vi "Synthetic_Jet_Per_Block.vi"() -> (5 "Plug in titles":string[](array[string]), 7 "Plug in values":string[](array[string]))   [LabVIEW 2011]
uses:
  Globals/Meas_global.vi
  Globals/Plug_in_data_global.vi
  <vilib>/Analysis/baseanly.llb/Scale 1D.vi
  <vilib>/Analysis/5stat.llb/RMS (DBL).vi
  <vilib>/Analysis/1siggen.llb/Ramp Pattern by Samples.vi
  <vilib>/Analysis/NI_AALBase.lvlib
  <vilib>/Analysis/NI_AALPro.lvlib
  <vilib>/Analysis/NI_AAL_SigProc.lvlib
panel:
  out "Max Current":dbl format="%0.2f"
  out "RMS Current":dbl format="%0.2f"
  out "RMS Power":dbl format="%0.2f"
  out "Current":dbl[](array[numeric])
  out "RV RMS Pressure":dbl format="%0.2f"
  out "Max Pressure":dbl format="%0.2f"
  out "RMS Dispacement":dbl format="%0.2f"
  out "Max Displacement":dbl format="%0.2f"
  out "Power":dbl[](array[numeric])
  out "Current Plot":cluster{dbl[], dbl[]}[](graph)
  out "RV Pressure":dbl[](array[numeric])=[-14.369666524328046, -57.77058962565634, -87.07652966541758, -117.51006835010423, -142.3114261743131, -158.09199483911908, -155.83679754926837, -151.8902022920296, -142.3114261743131, -120.32906496241762, -88.20412831034297, -49.31359978871612, -12.114469234477319, 29.02544421285115, 67.35217341201532, 101.7323073539407, 128.78305010385122, 147.3826153809706, 157.5310031852989, 162.59938472331393, 149.63781267082135, 136.11244129586606, 102.29610667640338, 72.99016663664214, 42.55081558780641, -5.354689729074237, -48.18600114379076, -84.25753305310417, -116.38246970517886, -138.36483091707433, -158.65579416158175, -165.41557366698484, -160.34719212896982, -149.0712056797162, -122.58426225226835, -92.71452289004439, -56.642990980730964, -17.188663136641456, 24.515049633149694, 61.15038086492581, 97.22191277423924, 132.1658460386273, 151.3292106382094, 160.34418743346322, 160.34418743346322, 155.27580589544817, 136.67624061832876, 106.80650125610484, 74.67575223988108, 33.5358387925526, -1.9718937942981463, -42.553820283313044, -85.38513169802953, -116.38246970517886, -141.74762685185044, -159.78339280650712, -164.28797502205947, -162.03859009635784, -141.18382752938774, -123.71186089719372, -94.40592085743245, -59.46198759304437, -20.007659748954865, 21.70186538498539, 58.3313842526124, 92.14771887207513, 124.27846788829885, 149.63781267082135, 160.34418743346322, 156.9672038628362, 155.27580589544817, 141.75043452049292, 110.18348482673184, 77.49474885219449, 41.987016265343726, 0.2833034955525799, -41.42622163838768, -76.37015490277572, -109.62269019977577, -131.59923904752216, -159.21959348404445, -167.67077095683558, -160.9109914514325, -151.8902022920296, -125.96705818704444, -102.29329900776088, -63.96656980859674, -33.53303112391013, 16.627671482821253, 53.82680203706004, 93.27531751700047, 122.58706992091082, 148.51021402589598, 158.65860183022428, 155.27580589544817, 156.9672038628362, 142.30842147880648, 120.3318726310601, 80.31374546450789, 48.18880881243323, 10.425878935731753, -34.6606297688355, -76.37015490277572, -108.49509155485042, -133.85443633737287, -151.8902022920296, -162.03859009635784, -164.28797502205947, -154.709198904343, -135.54583430476092, -104.54849629761163, -71.85976032307427, -32.96923180144745, 7.0430830009556615, 52.135404069672006, 85.95173868913471, 118.64047466367205, 142.30842147880648, 157.5310031852989, 159.78038811100052, 158.09480250776156, 142.30842147880648, 123.71466856583618, 86.5155380115974, 49.316407457358586, 13.244875548045162, -27.33705094096973, -69.04076371076087, -103.42089765268625, -130.4716404025968, -151.8902022920296, -160.34719212896982, -162.60238941882054, -154.14539958188033, -135.54583430476092, -104.54849629761163, -71.85976032307427, -36.91582705868622, 4.793698075254034, 51.007805424746635, 81.44134410943326, 115.82147805135864, 140.62283587556755, 154.1482072505228, 160.9079867559259, 156.40340454037351, 145.69121741358256, 120.89567195352278, 93.27531751700047, 54.95440068198541]
  out "RV Max Pressure":dbl format="%0.2f"
  out "Max Hot Wire":dbl
  in  "Ring":u16(ring) items=["Pressure", "Velocity"]
  out "RMS Hot Wire":dbl format="%0.2f"
  out "RMS Pressure":dbl format="%0.2f"
  out "Pressure v Frequency":cluster{dbl[], dbl[]}(graph)
  out "Pressure":cluster{dbl[], dbl[]}[](graph)
  out "Displacement":cluster{dbl[], dbl[]}[](graph)
  out "Hot Wire":cluster{dbl[], dbl[]}[](graph)
  out "Input Voltage":dbl[](array[numeric])=[-2.335942353515625, -4.445075804443359, -6.4589520715332025, -8.30833544555664, -9.929101578369139, -11.296158333740234, -12.468054029541014, -13.27053771972656, -13.752864338378906, -13.877860350341795, -13.706862088623046, -13.197119987792966, -12.333764633789063, -11.183243720703125, -9.745557248535155, -8.082506219482422, -6.230334830322265, -4.188578411865234, -2.067363562011719, 0.10821758300781249, 2.266141298828125, 4.396184863281249, 6.422607198486327, 8.238069721679688, 9.855583170166014, 11.26864217529297, 12.397788305664061, 13.200271995849608, 13.694680013427734, 13.847556176757811, 13.67051721557617, 13.127318933105467, 12.284873692626952, 11.125059395751952, 9.687837592773436, 8.003411781005859, 6.15077572265625, 4.139687470703125, 2.006391221923828, -0.14781514038085936, -2.321072939453125, -4.453904519042968, -6.44965868774414, -8.280919963378906, -9.916555510253906, -11.332867199707032, -12.452719946289061, -13.252415621337889, -13.737530255126952, -13.89923513305664, -13.710114772949218, -13.191079288330076, -12.333764633789063, -11.186031735839844, -9.7520626171875, -8.079718204345703, -6.215000747070311, -4.203912495117187, -2.088738344726562, 0.09613618408203123, 2.2508072155761716, 4.374810080566406, 6.367311564941406, 8.235281706542969, 9.874169937744139, 11.26864217529297, 12.38245422241211, 13.197483980712889, 13.700720712890623, 13.85638489135742, 13.661223831787108, 13.136147647705076, 12.263498909912107, 11.116230681152343, 9.681796893310546, 8.027574578857422, 6.160069106445311, 4.139687470703125, 2.021725305175781, -0.1357337414550781, -2.321072939453125, -4.426489036865234, -6.452911372070313, -8.280919963378906, -9.925848894042968, -11.308239732666014, -12.419263764648436, -13.261244335937498, -13.752864338378906, -13.914569216308593, -13.72544885620117, -13.182250573730467, -12.343058017578123, -11.198577803955077, -9.760891331787109, -8.107133686523436, -6.22382946166992, -4.215993894042969, -2.107325112304687, 0.08684280029296874, 2.2415138317871093, 4.365516696777344, 6.382645648193359, 8.207866224365233, 9.855583170166014, 11.222639925537107, 12.37966620727539, 13.200271995849608, 13.67655791503906, 13.841050808105468, 13.62451496582031, 13.118025549316405, 12.27279229370117, 11.131100095214844, 9.705959691162109, 8.048949361572266, 6.181443889160155, 4.1824370361328125, 2.040312072753906, -0.1357337414550781, -2.3024861718749996, -4.414407637939453, -6.422243205566406, -8.24142308227539, -9.907726795654296, -11.314280432128905, -12.452719946289061, -13.26449702026367, -13.746823638916014, -13.89923513305664, -13.700821389160156, -13.20037267211914, -12.357927431640622, -11.195325119628905, -9.733475849609373, -8.115962401123046, -6.245204244384766, -4.2220345935058585, -2.091991029052734, 0.08405478515624998, 2.226179748535156, 4.3473945983886715, 6.331067368164062, 8.19253214111328, 9.840249086914062, 11.237974008789063, 12.367120139160155, 13.182149897460938, 13.691891998291014, 13.828969409179685, 13.657971147460938, 13.139400332031247, 12.278832993164063, 11.131100095214844, 9.6971309765625, 8.048949361572266, 6.190272603759766, 4.161062253417969, 2.055181486816406, -0.11761164306640623, -2.284364073486328, -4.393032855224609, -6.410161806640624, -8.265585880126952, -9.916555510253906, -11.314280432128905, -12.431345163574218, -13.261244335937498, -13.761693052978515, -13.908528516845703, -13.716155472412108, -13.20641337158203, -12.343058017578123, -11.207406518554686, -9.785518798828125, -8.115962401123046, -6.2331228454589835, -4.23411599243164, -2.110113127441406, 0.05663930297851562, 2.2168863647460935, 4.35018261352539, 6.345936782226563, 8.19857284057617, 9.822126988525389, 11.241226693115234, 12.361079439697264, 13.227687478027343, 13.682598614501952, 13.838262792968749, 13.645889748535156, 13.136147647705076, 12.290914392089842, 11.143646163330077, 9.727334473876951, 8.027574578857422, 6.187484588623047, 4.176396336669922, 2.052393471679687, -0.1264403576660156, -2.2718180053710935, -4.389780170898437, -6.398080407714843, -8.24746378173828, -9.901221427001953, -11.308239732666014, -12.455972630615232, -13.246374921874999, -13.761693052978515, -13.89923513305664, -13.716155472412108, -13.20641337158203, -12.361180115966796, -11.207406518554686, -9.773437399902342, -8.119215085449218, -6.263791011962891, -4.252702760009765, -2.11661849609375, 0.0320118359375, 2.2140983496093747, 4.319979116210937, 6.339896082763671, 8.1804507421875, 9.843501771240234, 11.231933309326172, 12.364332124023436, 13.178897213134764, 13.688639313964844, 13.847556176757811, 13.636596364746092, 13.139400332031247, 12.306248475341796, 11.149686862792967, 9.721293774414061, 8.07357682861328, 6.220940770263671, 4.188477735595702, 2.0644748706054687, -0.09623686035156248, -2.2690299902343747, -4.389780170898437, -6.394827723388671, -8.244211097412109, -9.879846644287108, -11.302199033203124, -12.422051779785155, -13.252415621337889, -13.749611654052734, -13.902487817382811, -13.722196171874998, -13.20037267211914, -12.357927431640622, -11.186031735839844, -9.791559498291015, -8.115962401123046, -6.273084395751952, -4.2373686767578125, -2.1347405944824214, 0.041305219726562495, 2.208057650146484, 4.313473747558593, 6.3371080676269536, 8.167904674072265, 9.831420372314453, 11.235185993652344, 12.38245422241211, 13.197483980712889, 13.691891998291014, 13.835010108642576, 13.661223831787108, 13.15148173095703, 12.309036490478515, 11.158980246582031, 9.736627857666015, 8.085658227539062, 6.16889782104492, 4.209852518310547, 2.089102337646484, -0.09902487548828123, -2.262989290771484, -4.386992155761718, -6.394827723388671, -8.244211097412109, -9.879846644287108, -11.28082425048828, -12.428092479248045, -13.239869553222654, -13.73427757080078, -13.902487817382811, -13.73148955566406, -13.203625356445311, -12.370473499755859, -11.21669990234375, -9.797600197753905, -8.101092987060547, -6.281913110351562, -4.268036843261719, -2.128699895019531, 0.03526452026367187, 2.208057650146484, 4.316726431884765, 6.312480600585937, 8.155823275146483, 9.831420372314453, 11.241226693115234, 12.345745356445313, 13.166815814208983, 13.685386629638671, 13.853596876220703, 13.673305230712888, 13.148693715820311, 12.300207775878905, 11.155727562255858, 9.727334473876951, 8.113073709716796, 6.233022169189453, 4.213105202636719, 2.089102337646484, -0.0776500927734375, -2.2355738085937498, -4.374910756835937, -6.38274632446289, -8.222836314697265, -9.877058629150389, -11.296158333740234, -12.3918482824707, -13.243122237548828, -13.740318270263671, -13.914569216308593, -13.737530255126952, -13.20641337158203, -12.373261514892578, -11.244115384521482, -9.81618696533203, -8.149883251953124, -6.273084395751952, -4.240621361083984, -2.140781293945312, 0.02597113647460937, 2.1955115820312496, 4.29209896484375, 6.315733284912108, 8.159075959472656, 9.824915003662108, 11.201265142822265, 12.355038740234374, 13.176109197998045, 13.664476516113279, 13.835010108642576, 13.664476516113279, 13.160775114746093, 12.288126376953123, 11.16502094604492, 9.745921241455077, 8.094951611328124, 6.218152755126952, 4.23122730102539, 2.110477120361328, -0.08415546142578124, -2.2323211242675782, -4.362364688720703, -6.3613715417480465, -8.214007600097656, -9.861724545898436, -11.284076934814454, -12.413223065185546, -13.243122237548828, -13.755652353515623, -13.908528516845703, -13.722196171874998, -13.225000139160155, -12.370473499755859, -11.250156083984375, -9.82501567993164, -8.158711966552733, -6.303287893066406, -4.28615894165039, -2.186783543701172, 0.010637053222656246, 2.1746014685058594, 4.29209896484375, 6.294358502197265, 8.149782575683593, 9.76125532470703, 11.213811210937498, 12.361079439697264, 13.178897213134764, 13.673305230712888, 13.838262792968749, 13.673305230712888, 13.154734415283203, 12.321582558593748, 11.179890360107422, 9.748709256591797, 8.100992310791016, 6.242315552978514, 4.215893217773437, 2.1039717517089844, -0.0627806787109375, -2.2202397253417967, -4.328908507080078, -6.367412241210937, -8.161964650878906, -9.871017929687499, -11.265490167236328, -12.397888981933594, -13.233828853759764, -13.712902788085938, -13.908528516845703, -13.73427757080078, -13.218494770507812, -12.373261514892578, -11.238074685058592, -9.828268364257811, -8.168005350341796, -6.32187466064453, -4.28615894165039, -2.186783543701172, -0.016778428955078126, 2.159267385253906, 4.28327025024414, 6.309692585449218, 8.137701176757812, 9.797499521484374, 11.204517827148436, 12.3369166418457, 13.166815814208983, 13.67934593017578, 13.838262792968749, 13.661223831787108, 13.15752243041992, 12.321582558593748, 11.204517827148436, 9.77612473876953, 8.140489191894531, 6.220940770263671, 4.237268000488281, 2.1378926025390625, -0.05627531005859375, -2.2202397253417967, -4.3502832897949215, -6.343249443359374, -8.201461531982421, -9.861724545898436, -11.256196783447265, -12.397888981933594, -13.237081538085938, -13.749611654052734, -13.895982448730468, -13.728236871337888, -13.21245407104492, -12.38255489868164, -11.247368068847656, -9.861724545898436, -8.18938013305664, -6.309328592529297, -4.304281040039061, -2.177490159912109, -0.02003111328125, 2.1499740014648436, 4.258642783203125, 6.285065118408203, 8.13444849243164, 9.77612473876953, 11.195224443359375, 12.321582558593748, 13.182149897460938, 13.673305230712888, 13.822928709716795, 13.664476516113279, 13.172856513671874, 12.3369166418457, 11.22589260986328, 9.779377423095703, 8.113073709716796, 6.26973103515625, 4.261895467529296, 2.1499740014648436, -0.03211251220703125, -2.198864942626953, -4.328908507080078, -6.327915360107421, -8.171258034667968, -9.846390462646484, -11.268742851562498, -12.397888981933594, -13.221747454833983, -13.737530255126952, -13.895982448730468, -13.758905037841796, -13.237081538085938, -12.406717696533203, -11.262702152099608, -9.837561748046875, -8.186127448730469, -6.33674407470703, -4.313574423828125, -2.183530859375, -0.04140589599609375, 2.143933302001953, 4.255854768066406, 6.28181243408203, 8.125155108642577, 9.788670806884765, 11.179890360107422, 12.324370573730468, 13.15752243041992, 13.682598614501952, 13.85034419189453, 13.67051721557617, 13.163563129882812, 12.330411273193358, 11.201265142822265, 9.785418122558593, 8.125155108642577, 6.26694302001953, 4.264683482666015, 2.1467213171386716, -0.016778428955078126, -2.183530859375, -4.310786408691406, -6.327915360107421, -8.161964650878906, -9.828268364257811, -11.244115384521482, -12.38255489868164, -13.221747454833983, -13.72544885620117, -13.908528516845703, -13.706862088623046, -13.233828853759764, -12.400676997070313, -11.262702152099608, -9.852431162109374, -8.180086749267577, -6.33674407470703, -4.325655822753906, -2.208158326416015, -0.04140589599609375, 2.131851903076172, 4.261895467529296, 6.26694302001953, 8.137701176757812, 9.779377423095703, 11.192436428222656, 12.318329874267578, 13.170068498535155, 13.688639313964844, 13.838262792968749, 13.67655791503906, 13.172856513671874, 12.348998040771484, 11.210558526611328, 9.794711506347655, 8.13444849243164, 6.279024418945312, 4.28327025024414, 2.1653080847167967, -0.016778428955078126, -2.180278175048828, -4.304281040039061, -6.339996759033203, -8.161964650878906, -9.822227664794921, -11.238074685058592, -12.38255489868164, -13.215706755371093, -13.728236871337888, -13.89923513305664, -13.737530255126952, -13.243122237548828, -12.403929681396484, -11.277571566162107, -9.846390462646484, -8.18938013305664, -6.349290142822265, -4.353535974121093, -2.2295331091308594, -0.050234610595703125, 2.12859921875, 4.2800175659179684, 6.233022169189453, 8.103780325927733, 9.773336723632811, 11.192436428222656, 12.318329874267578, 13.160775114746093, 13.67655791503906, 13.847556176757811, 13.688639313964844, 13.184937912597654, 12.33970465698242, 11.204517827148436, 9.797499521484374, 8.146529891357421, 6.2911058178710935, 4.286058265380859, 2.1653080847167967, -0.013525744628906253, -2.1714494604492183, -4.28615894165039, -6.297247193603514, -8.168005350341796, -9.822227664794921, -11.22878130126953, -12.361180115966796, -13.203625356445311, -13.72544885620117, -13.917357231445312, -13.749611654052734, -13.218494770507812, -12.397888981933594, -11.256196783447265, -9.871017929687499, -8.214007600097656, -6.352078157958983, -4.328908507080078, -2.2230277404785155, -0.09623686035156248, 2.1039717517089844, 4.225186601562499, 6.2455682373046875, 8.094951611328124, 9.764043339843749, 11.16502094604492, 12.306248475341796, 13.15148173095703, 13.67051721557617, 13.84430349243164, 13.682598614501952, 13.184937912597654, 12.318329874267578, 11.231933309326172, 9.816086289062499, 8.161863974609375, 6.297146517333983, 4.2800175659179684, 2.2168863647460935, -0.026071812744140627, -2.162156076660156, -4.28615894165039, -6.291206494140624, -8.161964650878906, -9.81618696533203, -11.21995258666992, -12.373261514892578, -13.227788154296874, -13.740318270263671, -13.91131653198242, -13.737530255126952, -13.215706755371093, -12.419263764648436, -11.286864949951172, -9.861724545898436, -8.20750223144531, -6.364624226074218, -4.383739471435547, -2.2536959069824216, -0.07160939331054687, 2.0979310522460937, 4.200559134521484, 6.239527537841796, 8.079617528076172, 9.754749956054686, 11.16176826171875, 12.315541859130859, 13.139400332031247, 13.661223831787108, 13.826181394042967, 13.657971147460938, 13.188190596923828, 12.358291424560546, 11.231933309326172, 9.816086289062499, 8.173945373535155, 6.315733284912108, 4.313473747558593, 2.1927235668945313, 0.013889737548828125, -2.162156076660156, -4.270824858398437, -6.3004998779296875, -8.143842552490234, -9.803640897216797, -11.21995258666992, -12.373261514892578, -13.215706755371093, -13.716155472412108, -13.874607666015624, -13.73427757080078, -13.243122237548828, -12.413223065185546, -11.284076934814454, -9.879846644287108, -8.226088999023437, -6.38274632446289, -4.368405388183593, -2.2416145080566405, -0.07486207763671875, 2.0798089538574214, 4.207064503173828, 6.230234154052734, 8.06753612915039, 9.739880541992186, 11.16176826171875, 12.300207775878905, 13.160775114746093, 13.655183132324218, 13.838262792968749, 13.67934593017578, 13.182149897460938, 12.370372823486326, 11.207770511474608, 9.824915003662108, 8.161863974609375, 6.315733284912108, 4.316726431884765, 2.1955115820312496, 0.02271845214843749, -2.13148791015625, -4.258743459472656, -6.266579027099609, -8.13733718383789, -9.791559498291015, -11.210659202880858, -12.361180115966796, -13.246374921874999, -13.719408156738279, -13.895982448730468, -13.746823638916014, -13.246374921874999, -12.43459784790039, -11.292905649414063, -9.88914002807617, -8.25350448120117, -6.38274632446289, -4.383739471435547, -2.2657773059082027, -0.10831825927734373, 2.0798089538574214, 4.203811818847656, 6.21490007080078, 8.07357682861328, 9.733375173339843, 11.158980246582031, 12.32762325805664, 13.154734415283203, 13.661223831787108, 13.838262792968749, 13.682598614501952, 13.20352468017578, 12.370372823486326, 11.235185993652344, 9.818874304199218, 8.173945373535155, 6.32781468383789, 4.338101214599609, 2.2140983496093747, 0.05338661865234373, -2.1226591955566403, -4.249450075683593, -6.251709613037109, -8.119215085449218, -9.779478099365233, -11.213911887207031, -12.363968131103515, -13.20037267211914, -13.722196171874998, -13.89923513305664, -13.752864338378906, -13.246374921874999, -12.425304464111326, -11.311492416992186, -9.886352012939453, -8.24746378173828, -6.416202506103516, -4.389780170898437, -2.3057388562011716, -0.09902487548828123, 2.0677275549316403, 4.170355637207031, 6.196777972412109, 8.054990061035156, 9.730587158203125, 11.143646163330077, 12.306248475341796, 13.127318933105467, 13.664476516113279, 13.835010108642576, 13.691891998291014, 13.21235339477539, 12.364332124023436, 11.244014708251953, 9.852795155029296, 8.19857284057617, 6.345936782226563, 4.3441419140625, 2.2233917333984374, 0.04734591918945312, -2.1226591955566403, -4.243409376220702, -6.266579027099609, -8.107133686523436, -9.794812182617186, -11.213911887207031, -12.33655264892578, -13.197119987792966, -13.719408156738279, -13.91131653198242, -13.758905037841796, -13.237081538085938, -12.416011080322264, -11.302199033203124, -9.916555510253906, -8.250251796874998, -6.3613715417480465, -4.420448337402344, -2.2931927880859373, -0.1264403576660156, 2.0491407873535157, 4.17314365234375, 6.181443889160155, 8.052202045898436, 9.718505759277342, 11.140393479003905, 12.300207775878905, 13.133359632568357, 13.657971147460938, 13.862425590820312, 13.685386629638671, 13.160775114746093, 12.364332124023436, 11.247267392578124, 9.855583170166014, 8.161863974609375, 6.349189466552733, 4.334848530273437, 2.2382611474609373, 0.05942731811523437, -2.1040724279785157, -4.209953194580078, -6.248456928710937, -8.109921701660156, -9.760891331787109, -11.189284420166015, -12.349098717041013, -13.185038588867187, -13.722196171874998, -13.902487817382811, -13.758905037841796, -13.26449702026367, -12.422051779785155, -11.311492416992186, -9.919808194580078, -8.265585880126952, -6.428748574218749, -4.423701021728515, -2.2871520886230465, -0.1264403576660156, 2.052393471679687, 4.176396336669922, 6.172150505371094, 8.042908662109374, 9.70317167602539, 11.146434178466794, 12.284873692626952, 13.114772864990234, 13.643101733398437, 13.853596876220703, 13.688639313964844, 13.188190596923828, 12.373160838623045, 11.259348791503905, 9.849542470703124, 8.204613540039063, 6.367311564941406, 4.365516696777344, 2.2568479150390623, 0.07476140136718748, -2.0859503295898434, -4.2067005102539055, -6.2331228454589835, -8.107133686523436, -9.76693203125, -11.186031735839844, -12.318430550537107, -13.191079288330076, -13.722196171874998, -13.91131653198242, -13.746823638916014, -13.26449702026367, -12.440638547363282, -11.317533116455076, -9.929101578369139, -8.271626579589844, -6.428748574218749, -4.435782420654297, -2.2931927880859373, -0.14781514038085936, 2.0310186889648434, 4.155021553955078, 6.1628571215820305, 8.030827263183593, 9.693878292236327, 11.076269130859373, 12.263498909912107, 13.120813564453124, 13.655183132324218, 13.859637575683593, 13.688639313964844, 13.20352468017578, 12.370372823486326, 11.253308092041014, 9.861623869628906, 8.216694938964844, 6.367311564941406, 4.362264012451171, 2.2415138317871093, 0.09009548461914062, -2.082697645263672, -4.209953194580078, -6.22382946166992, -8.088546918945312, -9.730687834472656, -11.183243720703125, -12.321683234863281, -13.188291273193357, -13.712902788085938, -13.917357231445312, -13.752864338378906, -13.26728503540039, -12.446679246826172, -11.32682650024414, -9.94397099243164, -8.286960662841796, -6.440829973144531, -4.429741721191406, -2.321072939453125, -0.16036120849609373, 2.0189372900390623, 4.127606071777343, 6.156816422119141, 8.018281195068358, 9.70317167602539, 11.11297799682617, 12.269539609375, 13.127318933105467, 13.657971147460938, 13.85034419189453, 13.703973397216796, 13.197483980712889, 12.38245422241211, 11.256560776367186, 9.867664569091797, 8.238069721679688, 6.37985763305664, 4.365516696777344, 2.2568479150390623, 0.09009548461914062, -2.067363562011719, -4.182537712402343, -6.236375529785155, -8.073212835693358, -9.760891331787109, -11.171162321777343, -12.333764633789063, -13.182250573730467, -13.704074073486328, -13.91131653198242, -13.749611654052734, -13.26728503540039, -12.43459784790039, -11.335655214843749, -9.956517060546874, -8.302294746093748, -6.452911372070313, -4.445075804443359, -2.321072939453125, -0.16640190795898435, 1.9943098229980465, 4.133646771240234, 6.184231904296874, 8.024786563720703, 9.678544208984373, 11.11297799682617, 12.263498909912107, 13.127318933105467, 13.661223831787108, 13.838262792968749, 13.688639313964844, 13.20352468017578, 12.397788305664061, 11.277935559082032, 9.916454833984375, 8.256656489257812, 6.388686347656249, 4.386891479492187, 2.2721819982910154, 0.10821758300781249]
  out "Displacement":dbl[](array[numeric])=[-0.04333556876627609, -0.0421144060872396, -0.0457758823242187, -0.04516630688476564, -0.02685490209960939, -0.018920362386067757, -0.032349128255208304, -0.02990680289713543, -0.009764659993489633, -0.0030512829589843804, -0.006714770996093744, -0.011597409912109335, 0.017088848144531266, 0.014038959147135377, 0.01892159806315108, 0.01892159806315108, 0.03112718945312498, 0.038452153727213556, 0.03784257828776039, 0.03784257828776039, 0.03967331640625005, 0.04272521720377609, 0.04699626888020836, 0.040282891845703106, 0.02441381241861984, 0.031738776692708304, 0.031738776692708304, 0.02929645133463543, 0.003662094075520872, 0.003662094075520872, 0.006104419433593744, 0.0048832567545572525, -0.014649310709635377, -0.017089624267578096, -0.017699199707031266, -0.02441458854166667, -0.037231767171224006, -0.039672080729166614, -0.039672080729166614, -0.039062505289713556, -0.04150483064778643, -0.04882778312174474, -0.0457758823242187, -0.04516630688476564, -0.02868564021809894, -0.030518390136718754, -0.03173754101562498, -0.02624532666015622, -0.010376247233072955, -0.009155084554036463, -0.007933921874999972, -0.008545509114583294, 0.018310010823567757, 0.019531173502604138, 0.020140748942057307, 0.017088848144531266, 0.03417909025065102, 0.03600982836914057, 0.035400252929687515, 0.035400252929687515, 0.03967331640625005, 0.038452153727213556, 0.04089447908528643, 0.04272521720377609, 0.035400252929687515, 0.028686875895182262, 0.028686875895182262, 0.029908038574218754, 0.008544732991536463, 0.007935157552083294, 0.0030525186360677026, 0.003662094075520872, -0.02136268774414063, -0.018310786946614588, -0.01953194962565108, -0.017699199707031266, -0.04028366796875005, -0.0421144060872396, -0.040893243408203106, -0.039062505289713556, -0.04455471964518232, -0.04516630688476564, -0.0506585212402344, -0.04699704500325519, -0.02624532666015622, -0.02380300130208335, -0.02258385042317712, -0.030518390136718754, -0.012206985351562505, -0.007933921874999972, -0.008545509114583294, -0.0054936083170572525, 0.015258110026041716, 0.015869697265625038, 0.017700435384114588, 0.01892159806315108, 0.03600982836914057, 0.03600982836914057, 0.03112718945312498, 0.03600982836914057, 0.03784257828776039, 0.0415040545247396, 0.04089447908528643, 0.038452153727213556, 0.030517614013671923, 0.02075233618164063, 0.033569514811197965, 0.030517614013671923, 0.0030525186360677026, 0.0024409313964843804, -0.0030512829589843804, -0.0012205448404948305, -0.016480048828125038, -0.018310786946614588, -0.018920362386067757, -0.017089624267578096, -0.03662017993164057, -0.03173754101562498, -0.039062505289713556, -0.039672080729166614, -0.04516630688476564, -0.0457758823242187, -0.04516630688476564, -0.039672080729166614, -0.02807606477864588, -0.02807606477864588, -0.02868564021809894, -0.031127965576171923, -0.008545509114583294, -0.007933921874999972, -0.004272445638020872, -0.012206985351562505, 0.016479272705078096, 0.017700435384114588, 0.028686875895182262, 0.014648534586588546, 0.03417909025065102, 0.03600982836914057, 0.038452153727213556, 0.03967331640625005, 0.037230991048177065, 0.04089447908528643, 0.032959939371744795, 0.039061729166666614, 0.02746571321614588, 0.026856137776692712, 0.028686875895182262, 0.02929645133463543, 0.006104419433593744, 0.0024409313964843804, 0.0024409313964843804, 0.005492832194010422, -0.018920362386067757, -0.020141525065104138, -0.020141525065104138, -0.020751100504557307, -0.037231767171224006, -0.04333556876627609, -0.037231767171224006, -0.037231767171224006, -0.0421144060872396, -0.042723981526692656, -0.0457758823242187, -0.04699704500325519, -0.03173754101562498, -0.027466489339192712, -0.029297227457682262, -0.029297227457682262, -0.013428148030598996, -0.006714770996093744, -0.008545509114583294, -0.006714770996093744, 0.014038959147135377, 0.015258110026041716, 0.017700435384114588, 0.018310010823567757, 0.036621415608724006, 0.035400252929687515, 0.035400252929687515, 0.03417909025065102, 0.042113629964192656, 0.04089447908528643, 0.04272521720377609, 0.03784257828776039, 0.025025399658203162, 0.02929645133463543, 0.03234835213216147, 0.039061729166666614, 0.005492832194010422, 0.0030525186360677026, 0.0006101932779948305, 0.005492832194010422, -0.017089624267578096, -0.017089624267578096, -0.01953194962565108, -0.02380300130208335, -0.039672080729166614, -0.040893243408203106, -0.04028366796875005, -0.04333556876627609, -0.040893243408203106, -0.04699704500325519, -0.040893243408203106, -0.04333556876627609, -0.029297227457682262, -0.030518390136718754, -0.034179866373697965, -0.02685490209960939, -0.011597409912109335, -0.006714770996093744, -0.006103183756510422, -0.009764659993489633, 0.014038959147135377, 0.020140748942057307, 0.02258307430013018, 0.02075233618164063, 0.03112718945312498, 0.034790677490234345, 0.037230991048177065, 0.030517614013671923, 0.04089447908528643, 0.038452153727213556, 0.040282891845703106, 0.038452153727213556, 0.033569514811197965, 0.02807528865559894, 0.031738776692708304, 0.026856137776692712, 0.003662094075520872, 0.001831355957031211, -0.0054936083170572525, 6.178385416610865e-07, -0.014649310709635377, -0.017699199707031266, -0.01953194962565108, -0.017699199707031266, -0.035401029052734345, -0.04150483064778643, -0.040893243408203106, -0.03662017993164057, -0.04699704500325519, -0.0457758823242187, -0.04882778312174474, -0.04455471964518232, -0.030518390136718754, -0.02685490209960939, -0.02868564021809894, -0.030518390136718754, -0.010376247233072955, -0.006714770996093744, -0.006714770996093744, -0.008545509114583294, 0.015869697265625038, 0.02197349886067712, 0.020140748942057307, 0.02197349886067712, 0.03417909025065102, 0.039061729166666614, 0.03600982836914057, 0.036621415608724006, 0.03784257828776039, 0.038452153727213556, 0.036621415608724006, 0.036621415608724006, 0.03112718945312498, 0.03234835213216147, 0.031738776692708304, 0.032959939371744795, 0.0048832567545572525, 0.0006101932779948305, 0.0030525186360677026, 0.00427166951497393, -0.014649310709635377, -0.018310786946614588, -0.016480048828125038, -0.018920362386067757, -0.04516630688476564, -0.036010604492187515, -0.036010604492187515, -0.042723981526692656, -0.04760662044270836, -0.04760662044270836, -0.04882778312174474, -0.04638746956380213, -0.03173754101562498, -0.02990680289713543, -0.034179866373697965, -0.02685490209960939, -0.009764659993489633, -0.006714770996093744, -0.012206985351562505, -0.009764659993489633, 0.015869697265625038, 0.02075233618164063, 0.018310010823567757, 0.02563497509765622, 0.03600982836914057, 0.033569514811197965, 0.040282891845703106, 0.036621415608724006, 0.04333479264322915, 0.03784257828776039, 0.037230991048177065, 0.037230991048177065, 0.03417909025065102, 0.032959939371744795, 0.029908038574218754, 0.026856137776692712, 0.00427166951497393, 0.0067139948730469134, 0.003662094075520872, 0.003662094075520872, -0.018920362386067757, -0.02136268774414063, -0.020751100504557307, -0.013428148030598996, -0.03662017993164057, -0.04028366796875005, -0.040893243408203106, -0.04028366796875005, -0.039672080729166614, -0.0457758823242187, -0.04699704500325519, -0.04821820768229168, -0.031127965576171923, -0.03295870369466147, -0.02136268774414063, -0.02807606477864588, -0.010985822672526013, -0.012206985351562505, -0.012206985351562505, -0.0073243464355469134, 0.016479272705078096, 0.014038959147135377, 0.014648534586588546, 0.016479272705078096, 0.036621415608724006, 0.04455595532226564, 0.037230991048177065, 0.037230991048177065, 0.040282891845703106, 0.039061729166666614, 0.0415040545247396, 0.03600982836914057, 0.03234835213216147, 0.02258307430013018, 0.03112718945312498, 0.02807528865559894, 0.001831355957031211, -0.0006109694010416611, 0.0024409313964843804, 0.006104419433593744, -0.0219722631835938, -0.018310786946614588, -0.020141525065104138, -0.01953194962565108, -0.04150483064778643, -0.039062505289713556, -0.0421144060872396, -0.042723981526692656, -0.04455471964518232, -0.04394514420572915, -0.04516630688476564, -0.04394514420572915, -0.030518390136718754, -0.03295870369466147, -0.02868564021809894, -0.029297227457682262, -0.014037723470052055, -0.010376247233072955, -0.007933921874999972, -0.012206985351562505, 0.018310010823567757, 0.014648534586588546, 0.017700435384114588, 0.014648534586588546, 0.03234835213216147, 0.03600982836914057, 0.03112718945312498, 0.03784257828776039, 0.037230991048177065, 0.040282891845703106, 0.03784257828776039, 0.040282891845703106, 0.0213619116210938, 0.03112718945312498, 0.032959939371744795, 0.02807528865559894, 0.0048832567545572525, 0.0012197687174478888, 0.003662094075520872, 0.0006101932779948305, -0.016480048828125038, -0.02441458854166667, -0.018920362386067757, -0.01953194962565108, -0.036010604492187515, -0.04516630688476564, -0.04455471964518232, -0.0421144060872396, -0.04394514420572915, -0.04150483064778643, -0.04882778312174474, -0.037231767171224006, -0.035401029052734345, -0.025635751220703162, -0.02807606477864588, -0.02685490209960939, -0.006714770996093744, -0.011597409912109335, -0.007933921874999972, -0.007933921874999972, 0.017700435384114588, 0.016479272705078096, 0.016479272705078096, 0.014648534586588546, 0.03600982836914057, 0.038452153727213556, 0.035400252929687515, 0.03112718945312498, 0.038452153727213556, 0.037230991048177065, 0.04455595532226564, 0.038452153727213556, 0.030517614013671923, 0.02929645133463543, 0.02807528865559894, 0.030517614013671923, 0.007935157552083294, 0.0024409313964843804, -0.0006109694010416611, 6.178385416610865e-07, -0.016480048828125038, -0.014649310709635377, -0.016480048828125038, -0.014037723470052055, -0.04516630688476564, -0.04394514420572915, -0.032349128255208304, -0.04150483064778643, -0.04333556876627609, -0.04882778312174474, -0.04638746956380213, -0.04760662044270836, -0.029297227457682262, -0.02685490209960939, -0.030518390136718754, -0.030518390136718754, -0.013428148030598996, -0.0030512829589843804, -0.0073243464355469134, -0.0054936083170572525, 0.014648534586588546, 0.018310010823567757, 0.012817796468098996, 0.018310010823567757, 0.035400252929687515, 0.038452153727213556, 0.034790677490234345, 0.034790677490234345, 0.04272521720377609, 0.036621415608724006, 0.042113629964192656, 0.038452153727213556, 0.02624455053710939, 0.02746571321614588, 0.02563497509765622, 0.03234835213216147, 0.005492832194010422, -0.0018301202799478888, -0.0006109694010416611, 0.005492832194010422, -0.015258886149088546, -0.009764659993489633, -0.02258385042317712, -0.0219722631835938, -0.037231767171224006, -0.040893243408203106, -0.037841342610677065, -0.040893243408203106, -0.04333556876627609, -0.04638746956380213, -0.042723981526692656, -0.0421144060872396, -0.029297227457682262, -0.033570290934244795, -0.02990680289713543, -0.02807606477864588, -0.010376247233072955, -0.007933921874999972, -0.011597409912109335, -0.010376247233072955, 0.012817796468098996, 0.017700435384114588, 0.018310010823567757, 0.019531173502604138, 0.029908038574218754, 0.03784257828776039, 0.037230991048177065, 0.034790677490234345, 0.03784257828776039, 0.0415040545247396, 0.0415040545247396, 0.0415040545247396, 0.032959939371744795, 0.025025399658203162, 0.029908038574218754, 0.026856137776692712, 0.006104419433593744, 0.0030525186360677026, 0.0006101932779948305, -0.0012205448404948305, -0.015258886149088546, -0.017089624267578096, -0.018310786946614588, -0.02136268774414063, -0.039062505289713556, -0.0421144060872396, -0.039672080729166614, -0.03662017993164057, -0.04455471964518232, -0.0457758823242187, -0.04821820768229168, -0.040893243408203106, -0.030518390136718754, -0.025635751220703162, -0.027466489339192712, -0.02868564021809894, -0.010985822672526013, -0.008545509114583294, -0.0006109694010416611, -0.009764659993489633, 0.012817796468098996, 0.015258110026041716, 0.0213619116210938, 0.0213619116210938, 0.037230991048177065, 0.034790677490234345, 0.03600982836914057, 0.033569514811197965, 0.0415040545247396, 0.04333479264322915, 0.039061729166666614, 0.04089447908528643, 0.030517614013671923, 0.03234835213216147, 0.030517614013671923, 0.031738776692708304, 0.0067139948730469134, 6.178385416610865e-07, 0.0012197687174478888, 0.0006101932779948305, -0.013428148030598996, -0.018920362386067757, -0.01953194962565108, -0.02258385042317712, -0.03662017993164057, -0.039672080729166614, -0.037231767171224006, -0.04333556876627609, -0.04699704500325519, -0.04699704500325519, -0.04821820768229168, -0.0421144060872396, -0.03173754101562498, -0.030518390136718754, -0.031127965576171923, -0.02685490209960939, -0.009764659993489633, -0.0054936083170572525, -0.010985822672526013, -0.009764659993489633, 0.015869697265625038, 0.017088848144531266, 0.0213619116210938, 0.01892159806315108, 0.033569514811197965, 0.03234835213216147, 0.03600982836914057, 0.036621415608724006, 0.042113629964192656, 0.04577711800130213, 0.035400252929687515, 0.03784257828776039, 0.03112718945312498, 0.032959939371744795, 0.02807528865559894, 0.02807528865559894, 0.006104419433593744, 0.003662094075520872, 0.005492832194010422, 0.0067139948730469134, -0.018920362386067757, -0.0219722631835938, -0.02258385042317712, -0.018920362386067757, -0.03845292985026039, -0.0421144060872396, -0.04394514420572915, -0.04394514420572915, -0.04333556876627609, -0.04516630688476564, -0.04394514420572915, -0.0506585212402344, -0.03173754101562498, -0.029297227457682262, -0.02380300130208335, -0.025635751220703162, -0.012816560791015674, -0.010985822672526013, -0.010376247233072955, -0.002441707519531211, 0.017700435384114588, 0.025025399658203162, 0.014648534586588546, 0.017700435384114588, 0.03417909025065102, 0.042113629964192656, 0.037230991048177065, 0.02929645133463543, 0.038452153727213556, 0.038452153727213556, 0.04272521720377609, 0.039061729166666614, 0.032959939371744795, 0.02563497509765622, 0.02807528865559894, 0.028686875895182262, 0.007935157552083294, 0.0024409313964843804, 0.0030525186360677026, 0.00427166951497393, -0.02380300130208335, -0.014649310709635377, -0.015868461588541716, -0.016480048828125038, -0.04150483064778643, -0.0421144060872396, -0.03662017993164057, -0.0457758823242187, -0.04516630688476564, -0.04455471964518232, -0.04699704500325519, -0.04882778312174474, -0.02990680289713543, -0.02868564021809894, -0.02868564021809894, -0.033570290934244795, -0.012206985351562505, -0.010376247233072955, -0.0073243464355469134, -0.0018301202799478888, 0.015869697265625038, 0.017088848144531266, 0.019531173502604138, 0.02075233618164063, 0.03417909025065102, 0.032959939371744795, 0.030517614013671923, 0.036621415608724006, 0.039061729166666614, 0.03784257828776039, 0.04089447908528643, 0.038452153727213556, 0.03112718945312498, 0.02929645133463543, 0.029908038574218754, 0.02624455053710939, 0.006104419433593744, -0.0018301202799478888, -0.002441707519531211, 0.001831355957031211, -0.014649310709635377, -0.01953194962565108, -0.020141525065104138, -0.016480048828125038, -0.037841342610677065, -0.03845292985026039, -0.04150483064778643, -0.04150483064778643, -0.04821820768229168, -0.04394514420572915, -0.04821820768229168, -0.0457758823242187, -0.034179866373697965, -0.02807606477864588, -0.029297227457682262, -0.027466489339192712, -0.009764659993489633, -0.0030512829589843804, -0.006714770996093744, -0.009764659993489633, 0.017088848144531266, 0.018310010823567757, 0.01892159806315108, 0.017700435384114588, 0.03234835213216147, 0.039061729166666614, 0.039061729166666614, 0.036621415608724006, 0.034790677490234345, 0.03784257828776039, 0.0415040545247396, 0.03784257828776039, 0.02929645133463543, 0.030517614013671923, 0.026856137776692712, 0.03600982836914057, 0.0067139948730469134, 0.003662094075520872, 0.0012197687174478888, 0.0006101932779948305, -0.013428148030598996, -0.02258385042317712, -0.017699199707031266, -0.020751100504557307, -0.03845292985026039, -0.04028366796875005, -0.037231767171224006, -0.039672080729166614, -0.042723981526692656, -0.04394514420572915, -0.04394514420572915, -0.04638746956380213, -0.02868564021809894, -0.025635751220703162, -0.027466489339192712, -0.03478944181315102, -0.012206985351562505, -0.0054936083170572525, -0.006714770996093744, -0.006103183756510422, 0.011596633789062505, 0.017700435384114588, 0.01892159806315108, 0.017088848144531266, 0.035400252929687515, 0.03600982836914057, 0.03600982836914057, 0.03417909025065102, 0.04455595532226564, 0.04089447908528643, 0.04272521720377609, 0.03784257828776039, 0.031738776692708304, 0.030517614013671923, 0.037230991048177065, 0.03112718945312498, 0.005492832194010422, 0.0024409313964843804, 0.0024409313964843804, 0.007935157552083294, -0.012206985351562505, -0.017699199707031266, -0.025635751220703162, -0.018310786946614588, -0.04028366796875005, -0.036010604492187515, -0.040893243408203106, -0.037841342610677065, -0.0421144060872396, -0.04333556876627609, -0.04516630688476564, -0.0457758823242187, -0.02868564021809894, -0.030518390136718754, -0.02685490209960939, -0.02807606477864588, -0.014037723470052055, -0.009155084554036463, -0.010376247233072955, -0.007933921874999972, 0.015258110026041716, 0.015869697265625038, 0.0213619116210938, 0.017700435384114588, 0.02929645133463543, 0.038452153727213556, 0.02929645133463543, 0.036621415608724006, 0.037230991048177065, 0.04089447908528643, 0.039061729166666614, 0.04089447908528643, 0.031738776692708304, 0.026856137776692712, 0.029908038574218754, 0.02746571321614588, 0.009765895670572955, -0.0006109694010416611, 0.0048832567545572525, 0.0067139948730469134, -0.015868461588541716, -0.018310786946614588, -0.015868461588541716, -0.017699199707031266, -0.037841342610677065, -0.039062505289713556, -0.04028366796875005, -0.040893243408203106, -0.04760662044270836, -0.04943937036132817, -0.04882778312174474, -0.04455471964518232, -0.03173754101562498, -0.02807606477864588, -0.02624532666015622, -0.031127965576171923, -0.011597409912109335, -0.007933921874999972, -0.009764659993489633, -0.009764659993489633, 0.017088848144531266, 0.015258110026041716, 0.018310010823567757, 0.0213619116210938, 0.04272521720377609, 0.03417909025065102, 0.03417909025065102, 0.03600982836914057, 0.039061729166666614, 0.04333479264322915, 0.03600982836914057, 0.03784257828776039, 0.029908038574218754, 0.031738776692708304, 0.033569514811197965, 0.030517614013671923, 0.005492832194010422, 0.005492832194010422, 0.001831355957031211, -0.0006109694010416611, -0.015868461588541716, -0.018920362386067757, -0.017699199707031266, -0.02685490209960939, -0.03295870369466147, -0.0421144060872396, -0.037231767171224006, -0.04333556876627609, -0.04394514420572915, -0.04394514420572915, -0.0457758823242187, -0.04516630688476564, -0.03173754101562498, -0.02624532666015622, -0.02990680289713543, -0.02258385042317712, -0.011597409912109335, -0.006714770996093744, -0.012816560791015674, -0.009155084554036463, 0.012817796468098996, 0.01892159806315108, 0.015258110026041716, 0.018310010823567757, 0.032959939371744795, 0.032959939371744795, 0.042113629964192656, 0.038452153727213556, 0.04272521720377609, 0.040282891845703106, 0.039061729166666614, 0.038452153727213556, 0.031738776692708304, 0.031738776692708304, 0.030517614013671923, 0.02807528865559894, 0.0024409313964843804, 0.007935157552083294, 0.003662094075520872, 0.001831355957031211, -0.018920362386067757, -0.020751100504557307, -0.02136268774414063, -0.020141525065104138, -0.034179866373697965, -0.039062505289713556, -0.042723981526692656, -0.040893243408203106, -0.04028366796875005, -0.04150483064778643, -0.04516630688476564, -0.04943937036132817, -0.031127965576171923, -0.02807606477864588, -0.02624532666015622, -0.02807606477864588, -0.012206985351562505, -0.009155084554036463, -0.006714770996093744, -0.006103183756510422, 0.014038959147135377, 0.019531173502604138, 0.015258110026041716, 0.018310010823567757, 0.032959939371744795, 0.032959939371744795, 0.040282891845703106, 0.03600982836914057, 0.040282891845703106, 0.04089447908528643, 0.03784257828776039, 0.04089447908528643, 0.033569514811197965, 0.017088848144531266, 0.02807528865559894, 0.02807528865559894, 0.0067139948730469134, 0.0048832567545572525, 0.0030525186360677026, 0.0030525186360677026, -0.014649310709635377, -0.01953194962565108, -0.020141525065104138, -0.017699199707031266, -0.03845292985026039, -0.037231767171224006, -0.042723981526692656, -0.039672080729166614, -0.04516630688476564, -0.042723981526692656, -0.04394514420572915, -0.042723981526692656, -0.02502416398111984, -0.02868564021809894, -0.025635751220703162, -0.029297227457682262, -0.009155084554036463, -0.010985822672526013, -0.007933921874999972, -0.010376247233072955, 0.016479272705078096, 0.0213619116210938, 0.019531173502604138, 0.017088848144531266, 0.03112718945312498, 0.03600982836914057, 0.03600982836914057, 0.036621415608724006, 0.039061729166666614, 0.038452153727213556, 0.03784257828776039, 0.0415040545247396, 0.034790677490234345, 0.031738776692708304, 0.028686875895182262, 0.030517614013671923, 0.011596633789062505, 0.003662094075520872, 0.007935157552083294, 0.0012197687174478888, -0.015258886149088546, -0.0219722631835938, -0.015868461588541716, -0.018310786946614588, -0.034179866373697965, -0.0457758823242187, -0.04394514420572915, -0.04150483064778643, -0.039672080729166614, -0.040893243408203106, -0.04821820768229168, -0.04455471964518232, -0.03478944181315102, -0.02319342586263018, -0.027466489339192712, -0.02624532666015622, -0.012816560791015674, -0.009764659993489633, -0.009155084554036463, -0.00488202107747393, 0.017700435384114588, 0.018310010823567757, 0.017088848144531266, 0.017088848144531266, 0.036621415608724006, 0.038452153727213556, 0.040282891845703106, 0.03600982836914057, 0.039061729166666614, 0.036621415608724006, 0.0500481696777344, 0.042113629964192656, 0.031738776692708304, 0.030517614013671923, 0.030517614013671923, 0.03417909025065102, 0.010987058349609335, 0.0030525186360677026, 0.0030525186360677026, 0.00427166951497393, -0.013428148030598996, -0.016480048828125038, -0.010376247233072955, -0.012206985351562505, -0.03478944181315102, -0.03845292985026039, -0.039672080729166614, -0.04028366796875005]
  out "Pressure":dbl[](array[numeric])=[-14.369666524328046, -57.77058962565634, -87.07652966541758, -117.51006835010423, -142.3114261743131, -158.09199483911908, -155.83679754926837, -151.8902022920296, -142.3114261743131, -120.32906496241762, -88.20412831034297, -49.31359978871612, -12.114469234477319, 29.02544421285115, 67.35217341201532, 101.7323073539407, 128.78305010385122, 147.3826153809706, 157.5310031852989, 162.59938472331393, 149.63781267082135, 136.11244129586606, 102.29610667640338, 72.99016663664214, 42.55081558780641, -5.354689729074237, -48.18600114379076, -84.25753305310417, -116.38246970517886, -138.36483091707433, -158.65579416158175, -165.41557366698484, -160.34719212896982, -149.0712056797162, -122.58426225226835, -92.71452289004439, -56.642990980730964, -17.188663136641456, 24.515049633149694, 61.15038086492581, 97.22191277423924, 132.1658460386273, 151.3292106382094, 160.34418743346322, 160.34418743346322, 155.27580589544817, 136.67624061832876, 106.80650125610484, 74.67575223988108, 33.5358387925526, -1.9718937942981463, -42.553820283313044, -85.38513169802953, -116.38246970517886, -141.74762685185044, -159.78339280650712, -164.28797502205947, -162.03859009635784, -141.18382752938774, -123.71186089719372, -94.40592085743245, -59.46198759304437, -20.007659748954865, 21.70186538498539, 58.3313842526124, 92.14771887207513, 124.27846788829885, 149.63781267082135, 160.34418743346322, 156.9672038628362, 155.27580589544817, 141.75043452049292, 110.18348482673184, 77.49474885219449, 41.987016265343726, 0.2833034955525799, -41.42622163838768, -76.37015490277572, -109.62269019977577, -131.59923904752216, -159.21959348404445, -167.67077095683558, -160.9109914514325, -151.8902022920296, -125.96705818704444, -102.29329900776088, -63.96656980859674, -33.53303112391013, 16.627671482821253, 53.82680203706004, 93.27531751700047, 122.58706992091082, 148.51021402589598, 158.65860183022428, 155.27580589544817, 156.9672038628362, 142.30842147880648, 120.3318726310601, 80.31374546450789, 48.18880881243323, 10.425878935731753, -34.6606297688355, -76.37015490277572, -108.49509155485042, -133.85443633737287, -151.8902022920296, -162.03859009635784, -164.28797502205947, -154.709198904343, -135.54583430476092, -104.54849629761163, -71.85976032307427, -32.96923180144745, 7.0430830009556615, 52.135404069672006, 85.95173868913471, 118.64047466367205, 142.30842147880648, 157.5310031852989, 159.78038811100052, 158.09480250776156, 142.30842147880648, 123.71466856583618, 86.5155380115974, 49.316407457358586, 13.244875548045162, -27.33705094096973, -69.04076371076087, -103.42089765268625, -130.4716404025968, -151.8902022920296, -160.34719212896982, -162.60238941882054, -154.14539958188033, -135.54583430476092, -104.54849629761163, -71.85976032307427, -36.91582705868622, 4.793698075254034, 51.007805424746635, 81.44134410943326, 115.82147805135864, 140.62283587556755, 154.1482072505228, 160.9079867559259, 156.40340454037351, 145.69121741358256, 120.89567195352278, 93.27531751700047, 54.95440068198541]
  out "Zeros":dbl[](array[numeric])=[4.646586067783672e-05, 118.87402579240864, -0.31707763671875, 0.000152587890625]
  out "Results Files":path[](array[path])=[path "Z:/2012/Aero_Tunnel/Nick_Martin/Results_Post_Processed/Hc_50_Do_30_011_xls/2.8V/1000Hz_2.8V/HW (Uhw).txt", path "Z:/2012/Aero_Tunnel/Nick_Martin/Results_Post_Processed/Hc_50_Do_30_011_xls/2.8V/1000Hz_2.8V/Mano (Kulite).txt", path "Z:/2012/Aero_Tunnel/Nick_Martin/Results_Post_Processed/Hc_50_Do_30_011_xls/2.8V/1000Hz_2.8V/RV (Vdi).txt", path "Z:/2012/Aero_Tunnel/Nick_Martin/Results_Post_Processed/Hc_50_Do_30_011_xls/2.8V/1000Hz_2.8V/RV (Vin).txt", path "Z:/2012/Aero_Tunnel/Nick_Martin/Results_Post_Processed/Hc_50_Do_30_011_xls/2.8V/1000Hz_2.8V/Meta_data.txt"]
  out "Hotwire Velocity":dbl[](array[numeric])=[0.7024483807601632, 0.6675412456163817, 0.5895323110227707, 0.49031074204055786, 0.42691438865015513, 0.3394084814308287, 0.23578904568743037, 0.25366691174559236, 0.33295304653141033, 0.49209214943348795, 0.6883370982022367, 0.7438679491327939, 0.7488561162715902, 0.7589678895920078, 0.7192888185134453, 0.7488561162715902, 1.337540916483318, 2.219151729266594, 2.9544622748907425, 3.5404729498455514, 3.708339604593901, 3.7179336641835166, 3.3701554521077015, 2.9622337071163347, 2.391698738228721, 1.9105800263227906, 1.4423474355774917, 0.9888595719025276, 0.6766869435006765, 0.4445255792508789, 0.31416735538165336, 0.25987615369744704, 0.2640704220547692, 0.3539862894035718, 0.5248170019015588, 0.6450789258023775, 0.8031207268572089, 0.8661812309640644, 0.9273105691882173, 0.854953398802498, 0.6652475394112969, 0.5323501680682767, 0.4527208994149338, 0.3963947453513968, 0.3215735934400325, 0.2547002345865532, 0.20312396716143305, 0.19067373514148284, 0.19475184979504298, 0.2506085241538742, 0.38179629249318675, 0.5554086556113242, 0.7389073834362506, 0.7389073834362506, 0.4833101532037805, 0.4285029575259667, 0.8355107850701134, 1.7676820552614025, 2.711452127932239, 2.8765734176199724, 3.2918481520551097, 3.3790119382600463, 3.1565054732192617, 2.8232187477920423, 2.2755159061109453, 1.7986644990479717, 1.2934814970267474, 0.9213532354129534, 0.6019880848076496, 0.3890538759028031, 0.2609303028103791, 0.2109213101125532, 0.2516315571506584, 0.37610614593058017, 0.5957332168961281, 0.8521367036112985, 0.9333617784190384, 1.0176533377509658, 1.1012685828936268, 1.0570573140549384, 0.966977899142863, 0.8977808498943699, 0.7414097940340048, 0.6318871027591406, 0.515553298064717, 0.3890538759028031, 0.352629965631241, 0.3228304399946062, 0.37610614593058017, 0.5229762917068345, 0.6790133029944161, 0.9794134634820515, 1.094325029852917, 1.0671212533542318, 0.8949072204030958, 0.7339742967152022, 1.1221029336448058, 2.086338800352547, 3.4588620819465015, 3.6329070306398523, 4.1056812012643285, 4.178632225671737, 3.708339604593901, 3.2662622679871216, 2.7335045007128937, 2.0054329733935066, 1.5492738613700292, 1.0909374097783098, 0.7072543016720343, 0.4746583205726514, 0.3105174341660586, 0.25987615369744704, 0.2882210118660314, 0.4114204911141412, 0.6744144739020445, 0.9454374769804479, 1.1186439481693757, 1.333537615657161, 1.205298643836143, 1.2622098830890336, 1.0306275356337251, 0.8111325667744773, 0.6472691383298502, 0.5174103017798651, 0.41910820360114975, 0.3215735934400325, 0.27157824216369125, 0.2640704220547692, 0.32912351499823184, 0.4644318807231259, 0.6721011931605805, 0.9515867396099553, 1.3134236009313456, 1.333537615657161, 1.0570573140549384, 0.8493277181265805, 0.966977899142863, 1.5817354914083792, 2.689548589882659, 3.3438817739720115, 3.3352813677169024, 3.3005322187632617, 3.2490641045744786, 2.9465465235986277, 2.3719758567610105, 1.8458769214851825, 1.3870545291873828, 0.9424376601258055, 0.6472691383298502, 0.41296122170785327, 0.2962900372579463, 0.26513859115147165, 0.28936919397552724, 0.4285029575259667, 0.6883370982022367, 0.9731791768505899, 1.1221029336448058, 1.1978896834813806, 1.1721437018972554, 1.0470723984483417, 0.9036113734154885, 0.7717270435266773, 0.5875053805526903, 0.4175802991055394, 0.32912351499823184, 0.25987615369744704, 0.22444570228795369, 0.24859345843335884, 0.3278464496051216, 0.5100528808887389, 0.7872940142937261, 1.0570573140549384, 1.3173765963894182, 1.2934814970267474, 1.0306275356337251, 0.5957332168961281, 0.8747115557291242, 1.5631037700269614, 2.385199453504005, 3.1483100817117062, 3.549702286279565, 3.680070310143287, 3.531263700210581, 3.0500158736584235, 2.4516908455036446, 1.9939918245458867, 1.4165770122416856, 1.0470723984483417, 0.6790133029944161, 0.4160253197445939, 0.30334703669555324, 0.2516315571506584, 0.2825824098565621, 0.4332652721378527, 0.6836381107260541, 0.9303320867513544, 1.0772647179840713, 1.1186439481693757, 1.2468509650084403, 1.168556874546191, 1.1012685828936268, 0.9065686244371176, 0.7290181344283281, 0.5573837779518217, 0.41296122170785327, 0.3154002438500431, 0.25987615369744704, 0.2916532685761543, 0.3607764450664247, 0.5342571316118321, 0.7977798501922598, 0.9243586237765371, 1.1831099693509546, 1.3703549095730687, 1.6579238046286011, 1.614664069776915, 2.231660587227482, 2.868990309103322, 4.126384096851844, 4.064325082089164, 4.1892346918762176, 4.263425233993231, 3.892787046254057, 3.396601591606027, 2.763191575146408, 2.080539907073371, 1.614664069776915, 1.1433372832174988, 0.7290181344283281, 0.49031074204055786, 0.35939864066209243, 0.30215321701111547, 0.3446361536284674, 0.48857087063498766, 0.6539689717542287, 0.8718408959552219, 0.9794134634820515, 1.0638038107503998, 1.168556874546191, 1.1721437018972554, 1.0671212533542318, 0.8919816075681659, 0.7414097940340048, 0.6189197276629083, 0.4627338094250971, 0.37610614593058017, 0.35130549029480435, 0.3539862894035718, 0.43807130151439005, 0.5732713199849881, 0.8031207268572089, 1.0772647179840713, 1.1721437018972554, 0.7925225377155688, 0.7794782761854128, 0.805747474765305, 0.9243586237765371, 2.596430115893681, 3.0418866240942553, 3.756320214708898, 4.023527763449476, 3.8830199121551563, 3.387706548259113, 2.8765734176199724, 2.3983486690908404, 1.9270479090704316, 1.4208745275569028, 1.0372335933691093, 0.7414097940340048, 0.4780964230429739, 0.3875873292658822, 0.3265994199894102, 0.3875873292658822, 0.5978264186480753, 0.8718408959552219, 1.0874882120229405, 1.1831099693509546, 1.349779159026776, 1.3173765963894182, 1.2353950145458559, 1.1469331076514784, 1.0339261792224355, 0.8890639427077215, 0.7743213194485399, 0.5593647163893509, 0.37610614593058017, 0.28482218219237854, 0.25571583539044174, 0.2737457951690649, 0.4114204911141412, 0.5875053805526903, 0.8382817863237095, 1.205298643836143, 1.1612621081991399, 0.912446486068028, 1.0306275356337251, 1.4729352886874165, 2.62486936135211, 3.922621927188491, 4.274207561972722, 4.560351360286182, 4.328017230497862, 3.9427552581023746, 3.3177796438216056, 2.7042345822344904, 2.0629841917181353, 1.5355460261570675, 1.00474934633215, 0.6977182078065063, 0.49031074204055786, 0.3265994199894102, 0.27157824216369125, 0.28482218219237854, 0.38469764748903323, 0.5895323110227707, 0.8633918769858342, 0.9951771706382762, 1.0840480856856536, 1.1081773168966995, 1.1291926497439295, 1.0274046972022295, 0.8521367036112985, 0.6721011931605805, 0.5285917846367124, 0.4053670593755572, 0.2928127277345288, 0.2547002345865532, 0.2455856959565272, 0.3069026167783402, 0.47984101882015423, 0.6790133029944161, 0.8747115557291242, 1.0241233606506075, 1.043806862701397, 0.761526529660689, 0.4938789127526468, 0.9273105691882173, 2.0982200846655474, 3.066162042555621, 4.328017230497862, 5.093868275028248, 4.922565001155525, 4.22095938732302, 3.7179336641835166, 3.2067460936323435, 2.4248287284088708, 1.7472404874839633, 1.2165221163725108, 0.7743213194485399, 0.5064254361678288, 0.3380985111448663, 0.27923864136222437, 0.29052115108148824, 0.4412886748724451, 0.6953872944167402, 0.9036113734154885, 1.0739210745656957, 1.2429963481744597, 1.1941614395039473, 1.186809498908844, 1.0705166756548334, 0.9607460687507889, 0.6744144739020445, 0.4712055857207254, 0.34069578232766073, 0.2126810694687812, 0.16331774679676203, 0.1508980669461159, 0.19067373514148284, 0.35668397798543133, 0.6125192490317742, 0.8410604136003904, 1.1362466633649504, 1.2353950145458559, 0.9393835076959557, 0.7564163876044003, 1.2090557811764986, 2.345978984165183, 3.892787046254057, 4.4042580513721665, 4.5265019936942865, 4.349654684324991, 3.9127921514821664, 3.5404729498455514, 2.653420505288102, 2.237808811063759, 1.6872967177500737, 1.1794200368671366, 0.8218809910791918, 0.5418627984863992, 0.39490534088552987, 0.30932514089040103, 0.3539862894035718, 0.4974318207519951, 0.7640398890375952, 0.9607460687507889, 1.1116093771828468, 1.224026767625989, 1.2738721854209927, 1.1577030036880673, 1.0504147209150272, 0.8355107850701134, 0.6607262098829628, 0.5418627984863992, 0.33681932945705967, 0.2640704220547692, 0.20656549125032733, 0.19723645966664705, 0.2770352138433014, 0.3934205683086916, 0.6472691383298502, 1.0112173227747132, 1.201551223586451, 1.614664069776915, 1.0112173227747132, 0.7513864442198347, 0.9424376601258055, 2.139879499097569, 3.1982689269264353, 3.962768270355777, 4.560351360286182, 4.628686686587128, 4.274207561972722, 3.5404729498455514, 2.9386485073407305, 2.3072983680331554, 1.7270996412290098, 1.1326787299131487, 0.8031207268572089, 0.545699134600719, 0.3607764450664247, 0.2882210118660314, 0.30334703669555324, 0.4300964145642937, 0.6517599719214276, 0.9485079681794083, 1.0112173227747132, 1.1362466633649504, 1.1540791132828547, 1.0176533377509658, 0.9638577992708929, 0.7339742967152022, 0.5593647163893509, 0.38324469934599387, 0.25987615369744704, 0.20057830424903425, 0.14563810204732092, 0.14563810204732092, 0.20057830424903425, 0.3081119118995048, 0.48857087063498766, 0.7339742967152022, 0.912446486068028, 1.0604261023954136, 0.832803712855211, 0.4780964230429739, 0.8747115557291242, 2.080539907073371, 3.892787046254057, 3.9427552581023746, 4.437340294548773, 4.4042580513721665, 4.11591503406628, 3.595770290139124, 2.9309288398898734, 2.3072983680331554, 1.6971495809333512, 1.1978896834813806, 0.805747474765305, 0.49031074204055786, 0.31416735538165336, 0.2567560399587666, 0.24960970014090925, 0.38469764748903323, 0.5854421832404256, 0.832803712855211, 1.1012685828936268, 1.1941614395039473, 1.2545108677269579, 1.2738721854209927, 1.1398239380314752, 0.9546107246989661, 0.7438679491327939, 0.5573837779518217, 0.4237840399917169, 0.28482218219237854, 0.22537980333759153, 0.22910962467671195, 0.2837120161092538, 0.366274375677111, 0.4938789127526468, 0.6472691383298502, 0.7339742967152022, 0.7241399200628257, 0.4974318207519951, 0.3473021295730542, 0.6744144739020445, 2.0397293902267477, 2.689548589882659, 3.058163277776913, 3.387706548259113, 3.5404729498455514, 3.4055161640001548, 3.1565054732192617, 2.7042345822344904, 2.0746340794839053, 1.614664069776915, 1.1221029336448058, 0.7768696646912, 0.5046011541337854, 0.3265994199894102, 0.257799734674701, 0.2630274993313674, 0.3904949400288964, 0.5692749642798407, 0.7589678895920078, 0.9763243211625132, 1.0638038107503998, 1.0537659070747243, 1.0537659070747243, 0.9424376601258055, 0.753923862769211, 0.5998828089982506, 0.43487336506396945, 0.31416735538165336, 0.2144529190383808, 0.17504256787031672, 0.18350083559675717, 0.22723840125558117, 0.3718702757583549, 0.5732713199849881, 0.7414097940340048, 0.8355107850701134, 0.9700424557884636, 1.0874882120229405, 0.5895323110227707, 0.7266007763468763, 1.6872967177500737, 2.7780590252038326, 3.531263700210581, 3.8142213192738166, 4.054198795052426, 3.785277585405845, 3.2490641045744786, 2.830700640655069, 2.313751856029737, 1.6241624050646193, 1.186809498908844, 0.8111325667744773, 0.5118934656954126, 0.3190974727229169, 0.24064623728129034, 0.2662103247020581, 0.3539862894035718, 0.5672649801543218, 0.8004465909239399, 0.9607460687507889, 1.1612621081991399, 1.2127456833996888, 1.1221029336448058, 0.966977899142863, 0.8004465909239399, 0.6584519454346542, 0.5361306607199702, 0.3875873292658822, 0.2619663586208152, 0.17807172464563184, 0.1604827729524558, 0.18586665093554497, 0.2882210118660314, 0.4661351070634546, 0.62755470314993, 0.8465835178723983, 0.8437897445552671, 0.7463842873943493, 0.6232026769381256, 0.7846637059389331, 1.7070503448474328, 3.2747135952692794, 3.9127921514821664, 4.126384096851844, 4.22095938732302, 3.6894083808194824, 3.326520878398931, 2.838355490272179, 2.288158620187709, 1.667633598684049, 1.1649047423382997, 0.805747474765305, 0.5137395479786995, 0.3473021295730542, 0.26834246889750074, 0.2567560399587666, 0.36351681662534274, 0.5515158189185249, 0.8111325667744773, 0.9485079681794083, 1.0143979134109258, 1.0372335933691093, 0.9951771706382762, 0.9515867396099553, 0.805747474765305, 0.6584519454346542, 0.5064254361678288, 0.3621586135919258, 0.2704886919209304, 0.2630274993313674, 0.2759276123510148, 0.40838449647370145, 0.6019880848076496, 0.8661812309640644, 1.277806282896223, 1.8038005602326914, 1.9270479090704316, 1.00474934633215, 0.5672649801543218, 0.6766869435006765, 2.478800992225778, 4.095256150951129, 4.732797377408521, 5.143572896237162, 4.995415353781096, 4.617159923623934, 3.9526480013289853, 3.240668185916676, 2.5266687411982804, 1.9324877922664652, 1.2738721854209927, 0.8661812309640644, 0.5732713199849881, 0.3890538759028031, 0.29744068439217936, 0.28482218219237854, 0.4068579103639725, 0.6675412456163817, 0.9333617784190384, 1.094325029852917, 1.2856240102768004, 1.3457453866582445, 1.2353950145458559, 1.1012685828936268, 0.7925225377155688, 0.47984101882015423, 0.3215735934400325, 0.2348194817090447, 0.1874523139828738, 0.1563275804552501, 0.16260151891121147, 0.24960970014090925, 0.4285029575259667, 0.7463842873943493, 1.0504147209150272, 1.4640898593410148, 1.7120700315355377, 1.0909374097783098, 0.7463842873943493, 1.1012685828936268, 1.7371457360403002, 2.7262379329819586, 3.4769839689344937, 3.9729102246841053, 4.231433271064132, 3.8435516100202847, 3.2747135952692794, 2.7705403319186117, 2.104060052379086, 1.5723488696397285, 1.1256431502640345, 0.7640398890375952, 0.5028193824227155, 0.32912351499823184, 0.27264906754031537, 0.2619663586208152, 0.36351681662534274, 0.5936460933250521, 0.8084362986541932, 1.00474934633215, 1.1012685828936268, 1.1649047423382997, 1.0671212533542318, 0.9154277278078945, 0.7389073834362506, 0.5342571316118321, 0.3890538759028031, 0.23005970324589559, 0.15224756856105315, 0.1037448869380532, 0.0934089678064661, 0.1563275804552501, 0.3069026167783402, 0.5495978442800667, 0.761526529660689, 0.7899316367935779, 0.7488561162715902, 0.6859842672846472, 0.5010058677790397, 0.8977808498943699, 1.9270479090704316, 2.6750781291569243, 3.4142677751125463, 3.863344769603818, 3.9526480013289853, 3.8240440847825616, 3.326520878398931, 2.7409391400670002, 2.225398823185351, 1.577036362887818, 1.201551223586451, 0.753923862769211, 0.48680002799019134, 0.3420140618642725, 0.2609303028103791, 0.2770352138433014, 0.36907790474324076, 0.5361306607199702, 0.6977182078065063, 0.8804174436949216, 1.0241233606506075, 1.0671212533542318, 1.0638038107503998, 0.9454374769804479, 0.8031207268572089, 0.7048479433766429, 0.5613108799484567, 0.4543885084032831, 0.35668397798543133, 0.33037850108366873, 0.35939864066209243, 0.4527208994149338, 0.6495113367850958, 0.8111325667744773, 1.0772647179840713, 1.2738721854209927, 1.366270007107868, 0.9951771706382762, 0.5573837779518217, 0.6384547654690402, 1.1362466633649504, 2.3200882427441094, 3.3177796438216056, 3.756320214708898, 3.932677806051598, 3.8142213192738166, 3.3438817739720115, 2.785594760496306, 2.104060052379086, 1.633805890331584, 1.1151220502825987, 0.7414097940340048, 0.48155511778654714, 0.3278464496051216, 0.25366691174559236, 0.2567560399587666, 0.34069578232766073, 0.5495978442800667, 0.8465835178723983, 1.0504147209150272, 1.224026767625989, 1.2622098830890336, 1.1256431502640345, 0.9393835076959557, 0.7899316367935779, 0.4992346188095371, 0.366274375677111, 0.27923864136222437, 0.20142972081672816, 0.17056335002878986, 0.1874523139828738, 0.23578904568743037, 0.39935686362846146, 0.5732713199849881, 0.8218809910791918, 1.0274046972022295, 0.8493277181265805, 0.5712908463766779, 0.38179629249318675, 0.5998828089982506, 1.6725565314355326, 2.861266458807205, 3.531263700210581, 3.902778868104479, 3.932677806051598, 3.623688813029981, 3.115199012388799, 2.596430115893681, 2.127924578454152, 1.526481615309021, 1.0470723984483417, 0.7266007763468763, 0.439660968586301, 0.3069026167783402, 0.23578904568743037, 0.24960970014090925, 0.3718702757583549, 0.5593647163893509, 0.813781042811487, 0.9951771706382762, 1.1649047423382997, 1.1469331076514784, 1.0671212533542318, 0.9485079681794083, 0.7314927329350069, 0.5752989184529146, 0.4510922380517575, 0.3190974727229169, 0.24960970014090925, 0.2109213101125532, 0.19890159588543632, 0.2506085241538742, 0.366274375677111, 0.6146612080401536, 0.9333617784190384, 1.378726491578272, 2.104060052379086, 1.3870545291873828, 1.0176533377509658, 1.1362466633649504, 1.8942296626013952, 3.1565054732192617, 3.7369872620683817, 4.199642617163867, 4.3934269354381374, 3.962768270355777, 3.504129163584017, 2.838355490272179, 2.345978984165183, 1.7021449990480162, 1.201551223586451, 0.7463842873943493, 0.5118934656954126, 0.3190974727229169, 0.22723840125558117, 0.24859345843335884, 0.3446361536284674, 0.5515158189185249, 0.7768696646912, 0.9546107246989661, 1.0604261023954136, 1.1256431502640345, 1.0504147209150272, 0.9731791768505899, 0.7925225377155688, 0.5813756011128453, 0.3963947453513968, 0.2630274993313674, 0.20482994563832646, 0.1577026801155853, 0.1508980669461159, 0.20741996767698692, 0.3215735934400325, 0.4678085840096291, 0.6813462917423602, 0.7768696646912, 0.6883370982022367, 0.49209214943348795, 0.5248170019015588, 0.7564163876044003, 1.3954244010206769, 2.418254344571821, 2.9701846617031094, 3.240668185916676, 3.396601591606027, 3.1483100817117062, 2.8765734176199724, 2.391698738228721, 1.949112884533493, 1.4251828919600495, 1.0208507390615293, 0.6859842672846472, 0.4627338094250971, 0.3278464496051216, 0.2506085241538742, 0.27264906754031537, 0.37753668386881495, 0.5342571316118321, 0.7314927329350069, 0.8977808498943699, 0.9638577992708929, 1.0705166756548334, 1.1469331076514784, 1.0208507390615293, 0.8862135116635582, 0.7339742967152022, 0.5418627984863992, 0.3553191118608697, 0.23869755436944426, 0.21805173394386934, 0.2567560399587666, 0.4175802991055394, 0.6061737355194334, 0.7846637059389331, 0.9951771706382762, 1.0306275356337251, 0.8218809910791918, 0.6082972895862039, 0.5399333663691356, 0.883311529467325, 1.7070503448474328, 2.6606727674137813, 3.4410029919427765, 3.727548489055016, 3.698961440997273, 3.568031984171257, 3.0988371366193745, 2.7042345822344904, 2.0922724062914666, 1.5585456505096773, 1.104682847844109, 0.7414097940340048, 0.4938789127526468, 0.3253304562907996, 0.26513859115147165, 0.2630274993313674, 0.37753668386881495, 0.6517599719214276, 0.8521367036112985, 0.9393835076959557, 1.0112173227747132, 0.9607460687507889, 0.9213532354129534, 0.7794782761854128, 0.6340401241833241, 0.4974318207519951, 0.3446361536284674, 0.27157824216369125, 0.1758036258927378, 0.14180276389022875, 0.1437164911943332, 0.2109213101125532, 0.3240655696220858, 0.5772908959279709, 0.9095339098042275, 1.1186439481693757, 1.1540791132828547, 0.9333617784190384, 0.9036113734154885, 1.25063655381721, 1.7625268014029283, 2.915220472946987, 3.5222618363479614, 3.7179336641835166, 3.6894083808194824, 3.4858889343535586, 3.033940848579433, 2.4584797343278484, 2.02824331584618, 1.481734236157144, 1.0806869431492823, 0.6906483982222161, 0.449434651332473, 0.30572180563697204, 0.23578904568743037, 0.24064623728129034, 0.35130549029480435, 0.5854421832404256, 0.7846637059389331, 0.9888595719025276, 1.0570573140549384, 1.1012685828936268, 1.0874882120229405, 0.9983812634852319, 0.8633918769858342, 0.663006984543572, 0.5554086556113242, 0.4780964230429739, 0.4285029575259667, 0.34861411972597806, 0.3228304399946062, 0.3009632810428391, 0.3215735934400325, 0.3890538759028031, 0.5712908463766779, 0.8465835178723983, 1.0274046972022295, 0.9036113734154885, 0.7314927329350069, 1.2165221163725108, 2.21304632438833, 2.8232187477920423, 3.549702286279565, 3.698961440997273, 3.558762779213343, 3.531263700210581, 3.1316330588263854, 2.617698730858875, 2.086338800352547, 1.5174618142239407, 1.1398239380314752, 0.7414097940340048, 0.45938747581847156, 0.3215735934400325, 0.23966021705291574, 0.25263705146669396, 0.37045752141818683, 0.5936460933250521, 0.8218809910791918, 0.9546107246989661, 1.0840480856856536, 1.0739210745656957, 0.8919816075681659]
  out "AS Freq":dbl=40000.0 format="%.2f"
  out "Amplitude String":string="2.7500"
  out "Frequency String":string="1000"
  out "Amp":dbl=2.75 format="%.2f"
  out "Freq":dbl=1000.0 format="%.2f"
  # "You Must have selected the \"Save Data\" option on the \nMeasurement Program for this vi to work correctly"
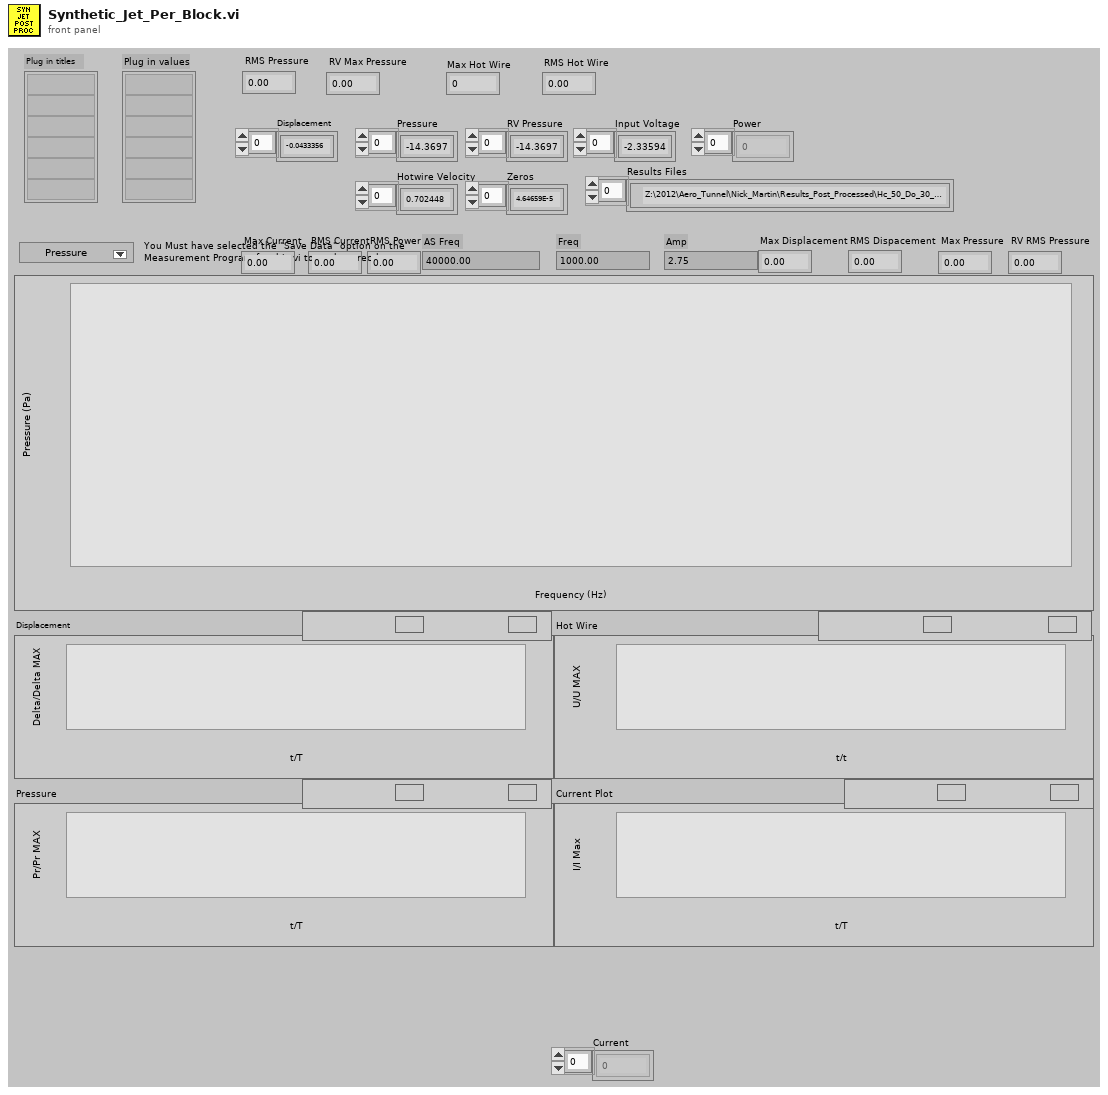
[diagram p1: front panel]
types:
  T1 = typedef "Analysis_info_cluster.ctl" = cluster{"Colour":u32, "Inst type":T2, "Inst name":string, "Symbol":string, "Code name":string, "Extra Info":string, "Inst Array":T3, "Index":i32, "Voltage Index":i32, "Extra Titles":string[], "Extra Values":string[]}
  T2 = typedef "Inst_type.ctl" = enum16{"Propeller anemometer", "Raw voltage", "Pressure Transducer", "Pitot-static tube", "Preston tube", "Hot wire", "Cross wire 1", "Cross wire 2", "Generic Linear", "Generic Polynomial", "Generic BackPoly", "Fast FID", "Thermocouple", "Cold wire", "Pulsed Wire", "LDA Vel", "LDA Tran time", "LDA Arr time"}
  T3 = typedef "Instrument_Array.ctl" = enum16{"PWA", "LDA", "Analogue"}
  T4 = cluster{"Name":string, "X":dbl, "Y":dbl, "Z":dbl}[]
  T5 = cluster{"Name":string, "X":dbl, "Y":dbl, "Z":dbl}
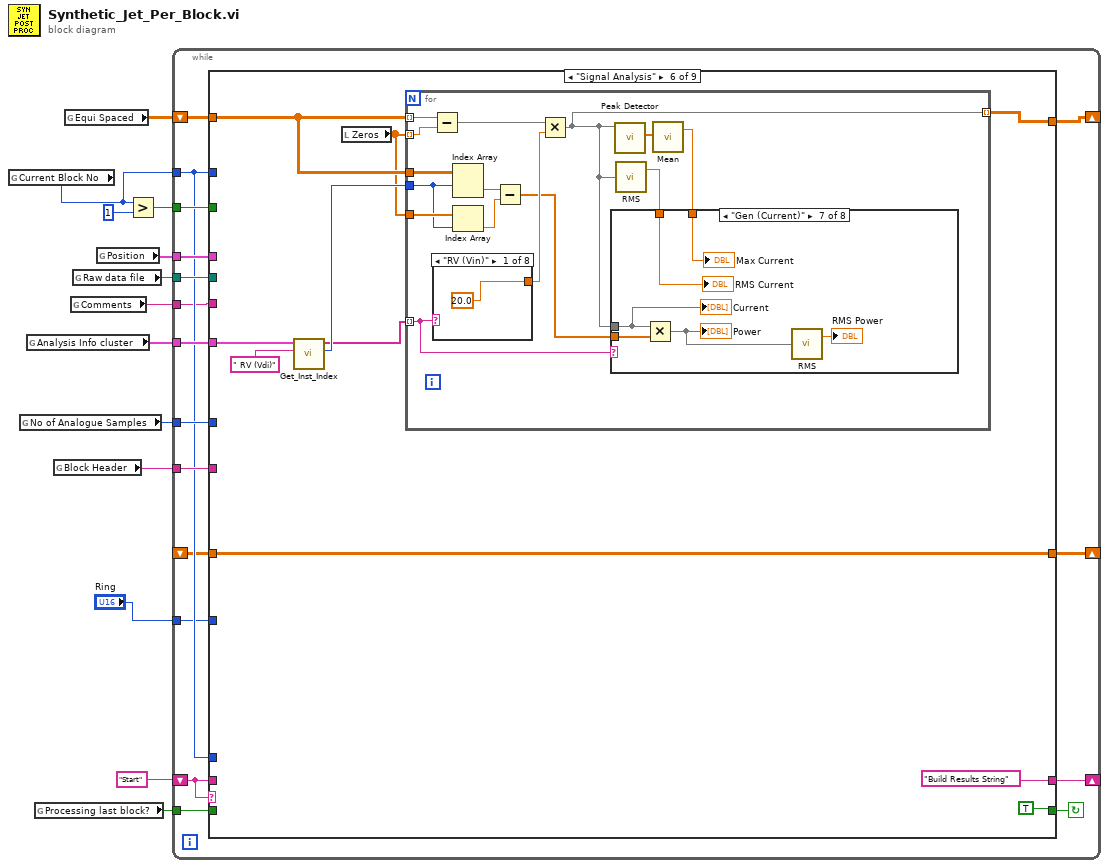
[diagram p0: block diagram]
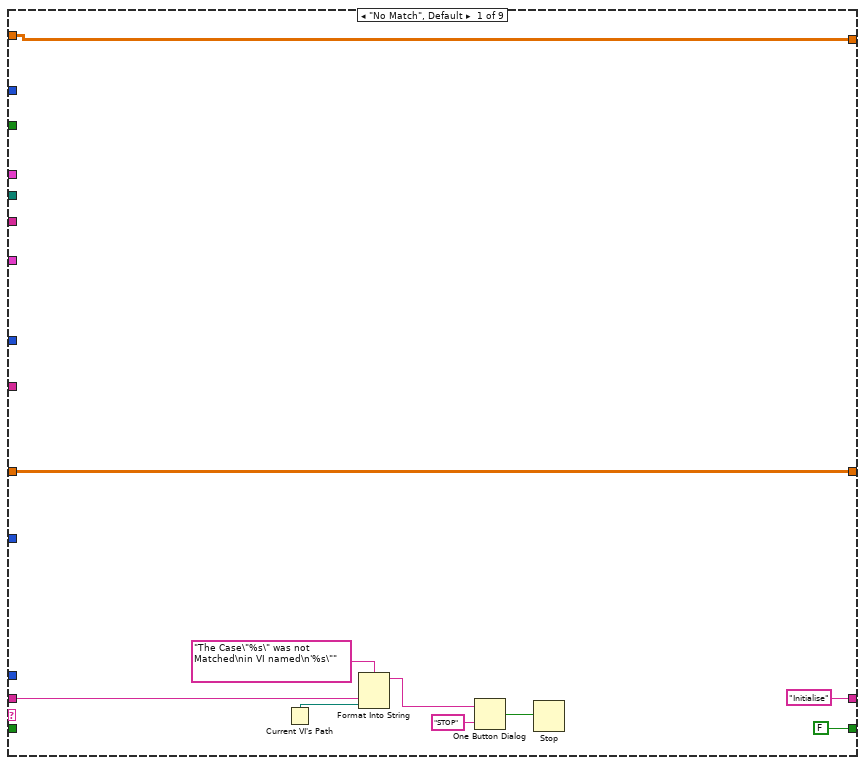
[diagram p2: hidden frame]
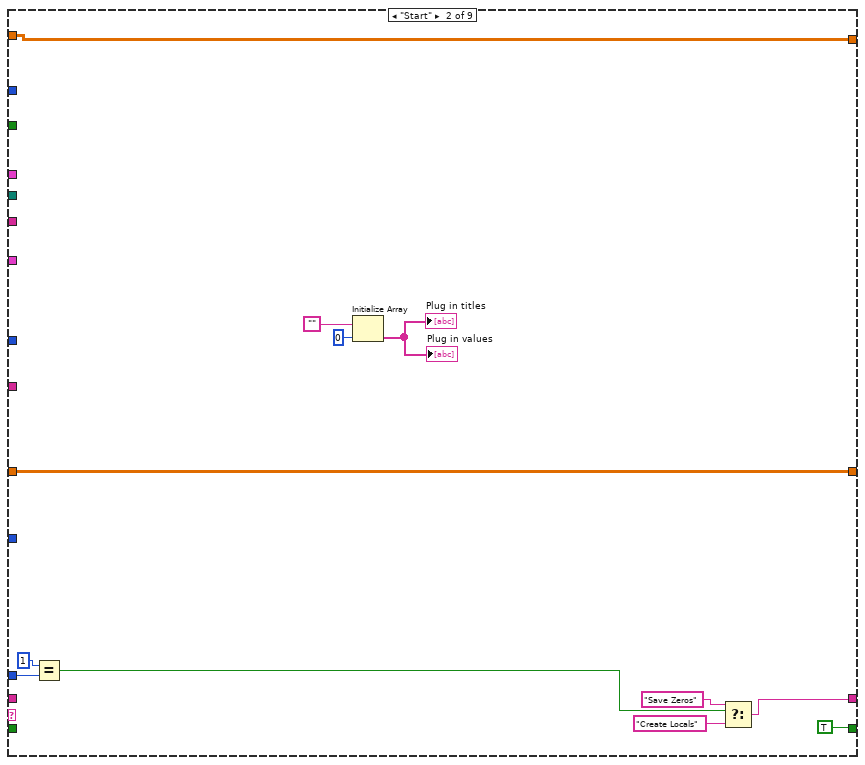
[diagram p3: hidden frame]
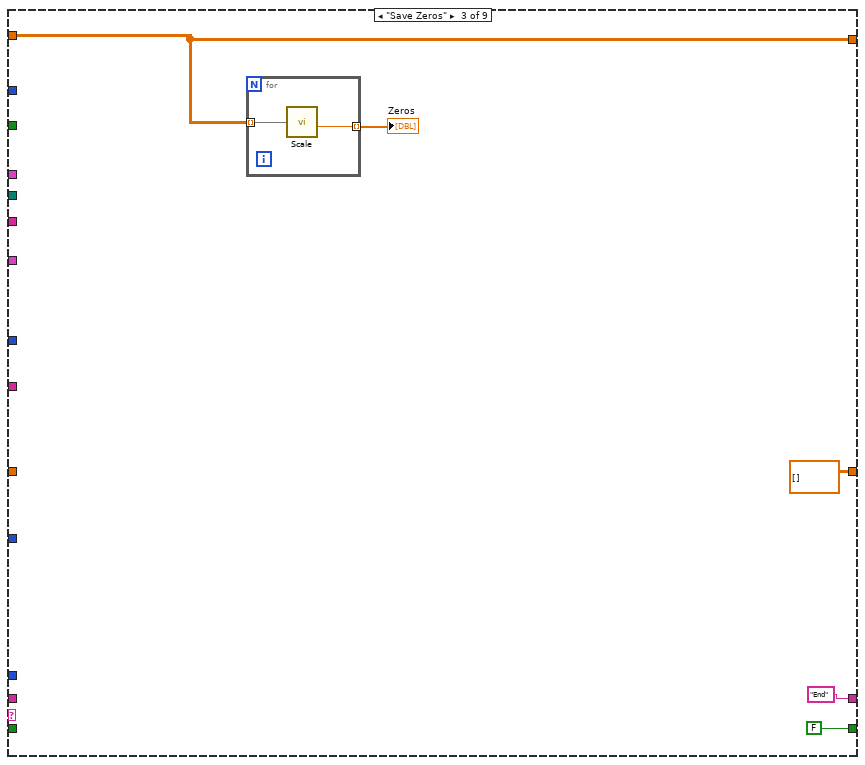
[diagram p4: hidden frame]
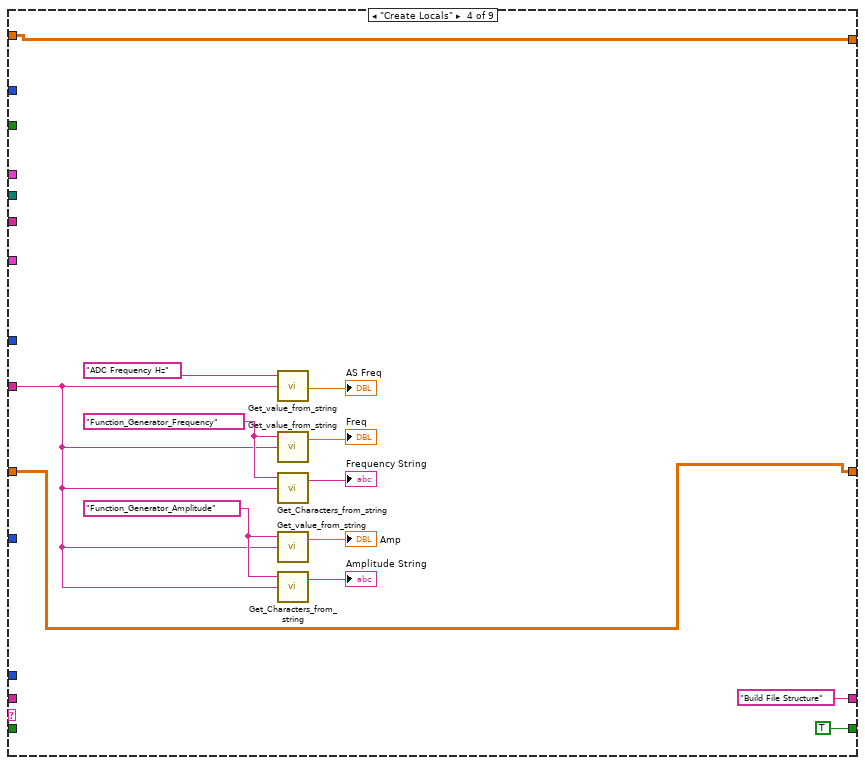
[diagram p5: hidden frame]
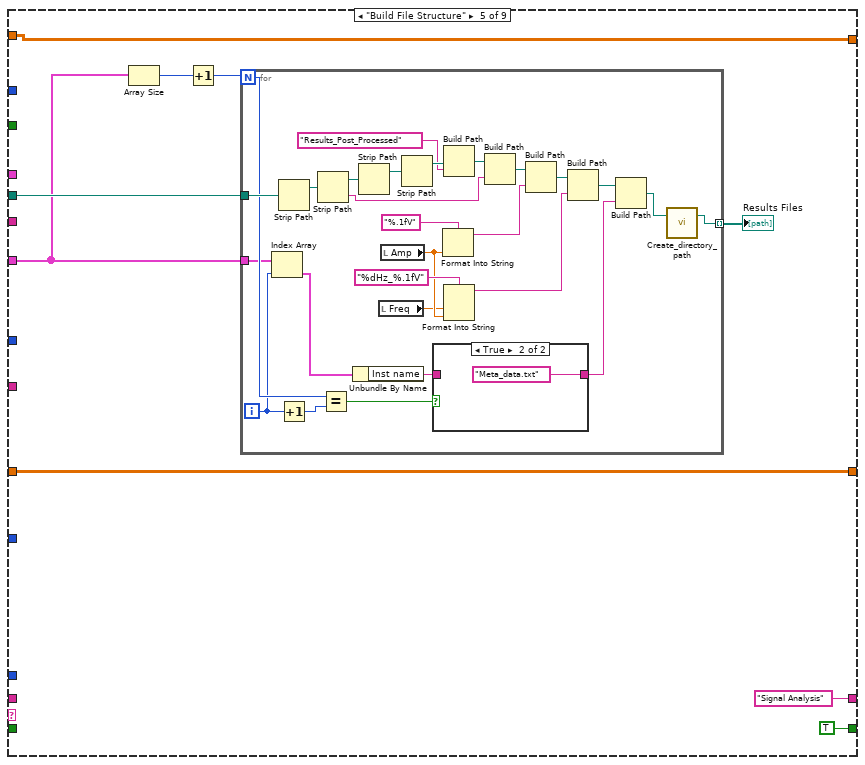
[diagram p6: hidden frame]
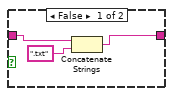
[diagram p7: hidden frame]
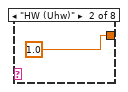
[diagram p8: hidden frame]
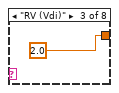
[diagram p9: hidden frame]
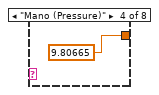
[diagram p10: hidden frame]
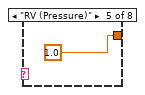
[diagram p11: hidden frame]
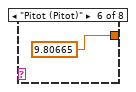
[diagram p12: hidden frame]
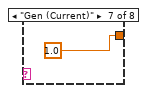
[diagram p13: hidden frame]
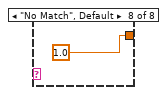
[diagram p14: hidden frame]
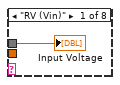
[diagram p15: hidden frame]
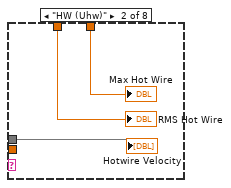
[diagram p16: hidden frame]
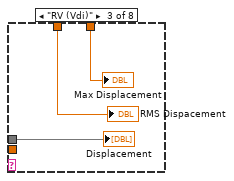
[diagram p17: hidden frame]
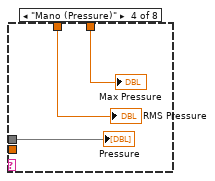
[diagram p18: hidden frame]
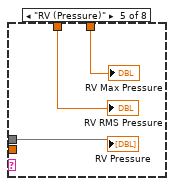
[diagram p19: hidden frame]
diagram:
  n1 = global read "Meas_global.vi" "Current Block No"() -> (w9:i32)
  n2 = global read "Meas_global.vi" "No of Analogue Samples"() -> (w5:i32)
  n3 = global read "Meas_global.vi" "Analysis Info cluster"() -> (w8:T1[])
  n4 = global read "Meas_global.vi" "Processing last block?"() -> (w3:bool)
  n5 = global read "Plug_in_data_global.vi" "Block Header"() -> (w6:string)
  n6 = global read "Plug_in_data_global.vi" "Equi Spaced"() -> (w7:dbl[][])
  n7 = global read "Meas_global.vi" "Comments"() -> (w1:string)
  n8 = global read "Meas_global.vi" "Raw data file"() -> (w12:path)
  n9 = global read "Meas_global.vi" "Position"() -> (w4:T4)
  n10 = Greater?(x=w9, y=1) -> (0:w10:bool)
  n11 = while {
    shift-left: "Start" -> [w30]
    shift-right: [w20] -> _
    tunnel: w12 -> [w29]
    tunnel: w10 -> [w28]
    tunnel: w9 -> [w21]
    tunnel: w8 -> [w27]
    tunnel: w6 -> [w25]
    tunnel: w5 -> [w24]
    tunnel: w4 -> [w23]
    tunnel: w3 -> [w22]
    shift-right: [w18] -> _
    shift-left: w7 -> [w26]
    shift-right: [w17] -> _
    shift-left: _ -> [w16]
    tunnel: "Ring" -> [w15]
    tunnel: w1 -> [w14]
    stop <- w19 continue-if-true
    n12 = case shown="\"Signal Analysis\"" w30 {
      tunnel: w30 -> [w36 _ _ _ _ _ _ _ _]
      tunnel: w29 -> [_ _ _ _ w81 _ w174 _ w299]
      tunnel: w28 -> [_ _ _ _ _ _ _ _ _]
      tunnel: w21 -> [_ _ _ _ _ _ _ _ _]
      tunnel: w27 -> [_ _ _ _ w76 w118 _ _ _]
      tunnel: w26 -> [w32 w42 w54 w61 w74 w116 w170 w253 w305]
      tunnel: w25 -> [_ _ _ w67 _ _ _ _ _]
      tunnel: w24 -> [_ _ _ _ _ _ _ w277 _]
      tunnel: w23 -> [_ _ _ _ _ _ w175 _ _]
      tunnel: w22 -> [_ _ _ _ _ _ _ w278 _]
      tunnel: w21 -> [_ w49 _ _ _ _ _ _ _]
      tunnel: ["Initialise" w44 "End" ("t") "Build File Structure" "Signal Analysis" "Build Results String" "Plot Data" "End" "End"] -> w20
      tunnel: [FALSE TRUE FALSE TRUE TRUE TRUE TRUE ("Processing last block?") w278 FALSE ("Processing last block?")] -> w19
      tunnel: [w32 w42 w54 w61 w74 w119 w170 w253 w305] -> w18
      tunnel: [w31 w41 dbl[][] [] w60 w73 w121 w169 w247 w290] -> w17
      tunnel: w16 -> [w31 w41 _ w60 w73 w121 w169 w248 w290]
      tunnel: w15 -> [_ _ _ _ _ _ _ w240 _]
      tunnel: w14 -> [_ _ _ _ _ _ w168 _ w284]
      frame "No Match", Default {
        n13 = Current VI's Path() -> (path=w35:path)
        n14 = Format Into String(format string="The Case\"%s\" was not Matched\nin VI named\n'%s\"" ("Format String"), w36, w35) -> (resulting string=w39:string)  [unwired: 2 in, 1 out]
        n15 = One Button Dialog(message=w39, button name ("OK")="STOP") -> (true=w37:bool)
        n16 = Stop(stop? (T)=w37) -> ()
      }
      frame "Start" {
        n17 = Equal?(x=1, y=w49) -> (x = y?=w47:bool)
        n18 = Initialize Array("", 0) -> (→"Plug in values" →"Plug in titles":string[])
        n19 = Select(t="Save Zeros", s=w47, f="Create Locals") -> (s? t:f=w44:string)
      }
      frame "Save Zeros" {
        (unwired) FALSE ("Processing last block?")
        (unwired) "End" ("t")
        (unwired) "End" ("t")
        (unwired) FALSE ("Processing last block?")
        n20 = for {
          tunnel: w54 -> [w59] mode=indexing
          tunnel: [w58] -> w56 mode=indexing
          n21 = call-poly <vilib>:"Scale.vi"("X"=w59) -> ("offset"=w58:dbl)  [unwired: 3 out]
        }
        "Zeros" <- w56
      }
      frame "Create Locals" {
        w69 = "Function_Generator_Amplitude" ("Variable name")
        w70 = "Function_Generator_Frequency" ("Variable name")
        n22 = call "Get_value_from_string.vi"("Input string"=w67, "Variable name"="ADC Frequency Hz") -> ("Value"=→"AS Freq":dbl)  [unwired: 1 in, 1 out]
        n23 = call "Get_value_from_string.vi"("Input string"=w67, "Variable name"=w70) -> ("Value"=→"Freq":dbl)  [unwired: 1 in, 1 out]
        n24 = call "Get_Characters_from_string.vi"("Input string"=w67, "Variable name"=w70) -> ("Value"=→"Frequency String":string)  [unwired: 1 in, 1 out]
        n25 = call "Get_value_from_string.vi"("Input string"=w67, "Variable name"=w69) -> ("Value"=→"Amp":dbl)  [unwired: 1 in, 1 out]
        n26 = call "Get_Characters_from_string.vi"("Input string"=w67, "Variable name"=w69) -> ("Value"=→"Amplitude String":string)  [unwired: 1 in, 1 out]
      }
      frame "Build File Structure" {
        n27 = Array Size(array=w76) -> (size(s)=w75:i32)
        n28 = Increment(x=w75) -> (x+1=w79:i32)
        n29 = for {
          N: w79 -> [w90]
          tunnel: w81 -> [w99]
          tunnel: [w98] -> w80 mode=indexing
          tunnel: w76 -> [w84]
          i -> [w82]
          n30 = Index Array(array=w84, index=w82) -> (element=w83:T1)
          n31 = Strip Path(path=w99) -> (stripped path=w108:path)  [unwired: 1 out]
          n32 = Increment(x=w82) -> (x+1=w85:i32)
          n33 = Strip Path(path=w108) -> (stripped path=w106:path, name=w102:string)
          n34 = Equal?(x=w90, y=w85) -> (x = y?=w88:bool)
          n35 = Unbundle By Name(w83) -> ("Inst name"=w87:string)
          n36 = Strip Path(path=w106) -> (stripped path=w107:path)  [unwired: 1 out]
          n37 = local read "Freq"() -> (w93:dbl)
          n38 = local read "Amp"() -> (w94:dbl)
          n39 = Strip Path(path=w107) -> (stripped path=w105:path)  [unwired: 1 out]
          n40 = case shown="True" w88 {
            tunnel: w87 -> [w111 _]
            tunnel: [w109 "Meta_data.txt"] -> w86
            frame False {
              n41 = Concatenate Strings(w111, ".txt" ("string")) -> (w109:string)
            }
            frame True {
            }
          }
          n42 = Format Into String(format string="%.1fV", w94) -> (resulting string=w96:string)  [unwired: 2 in, 1 out]
          n43 = Build Path(base path=w105, name or relative path="Results_Post_Processed") -> (appended path=w103:path)
          n44 = Format Into String(format string="%dHz_%.1fV", w93, w94) -> (resulting string=w92:string)  [unwired: 2 in, 1 out]
          n45 = Build Path(base path=w103, name or relative path=w102) -> (appended path=w101:path)
          n46 = Build Path(base path=w101, name or relative path=w96) -> (appended path=w100:path)
          n47 = Build Path(base path=w100, name or relative path=w92) -> (appended path=w91:path)
          n48 = Build Path(base path=w91, name or relative path=w86) -> (appended path=w89:path)
          n49 = call "Create_directory_path.vi"("Path name"=w89) -> ("Path name Out"=w98:path)  [unwired: 1 in, 1 out]
        }
        "Results Files" <- w80
      }
      frame "Signal Analysis" {
        n50 = call "Get_Inst_Index.vi"("Inst name search"=" RV (Vdi)" ("element"), "Analysis Info cluster"=w118) -> ("Index of Instance"=w115:i32, "Inst Name Array"=w114:string[])  [unwired: 8 in]
        n51 = local read "Zeros"() -> (w113:dbl[])
        n52 = for {
          tunnel: w116 -> [w137] mode=indexing
          tunnel: w113 -> [w136] mode=indexing
          tunnel: [w125] -> w119 mode=indexing
          tunnel: w116 -> [w132]
          tunnel: w115 -> [w129]
          tunnel: w114 -> [w131] mode=indexing
          tunnel: w113 -> [w130]
          n53 = Subtract(x=w137, y=w136) -> (x-y=w135:dbl[])
          n54 = case shown="\"RV (Vin)\"" w131 {
            tunnel: [20.0 1.0 2.0 9.80665 1.0 9.80665 1.0 1.0] -> w134
            frame "RV (Vin)" {
            }
            frame "HW (Uhw)" {
            }
            frame "RV (Vdi)" {
            }
            frame "Mano (Pressure)" {
            }
            frame "RV (Pressure)" {
            }
            frame "Pitot (Pitot)" {
            }
            frame "Gen (Current)" {
            }
            frame "No Match", Default {
            }
          }
          n55 = Index Array(array=w132, index (row)=w129) -> (element=w128:dbl[])  [unwired: 1 in]
          n56 = Index Array(array=w130, index=w129) -> (element=w127:dbl)
          n57 = Subtract(x=w128, y=w127) -> (x-y=w126:dbl[])
          n58 = Multiply(x=w135, y=w134) -> (x*y=w125:dbl[])
          n59 = call <vilib>:"Peak Detector.vi"("X"=w125) -> ("Amplitudes"=w133:dbl[])  [unwired: 6 in, 4 out]
          n60 = call-poly <vilib>:"RMS.vi"("X"=w125) -> ("rms value"=w124:dbl)  [unwired: 1 out]
          n61 = call <vilib>:"Mean.vi"("X"=w133) -> ("mean"=w123:dbl)  [unwired: 1 out]
          n62 = case shown="\"Gen (Current)\"" w131 {
            tunnel: w125 -> [w146 w149 w152 w155 w158 _ w163 _]
            tunnel: w126 -> [_ _ _ _ _ _ w164 _]
            tunnel: w124 -> [_ w148 w151 w153 w156 _ w160 _]
            tunnel: w123 -> [_ w147 w150 w154 w157 _ w159 _]
            frame "RV (Vin)" {
              "Input Voltage" <- w146
            }
            frame "HW (Uhw)" {
              "Hotwire Velocity" <- w149
              "RMS Hot Wire" <- w148
              "Max Hot Wire" <- w147
            }
            frame "RV (Vdi)" {
              "Displacement" <- w152
              "Max Displacement" <- w150
              "RMS Dispacement" <- w151
            }
            frame "Mano (Pressure)" {
              "Pressure" <- w155
              "RMS Pressure" <- w153
              "Max Pressure" <- w154
            }
            frame "RV (Pressure)" {
              "RV Pressure" <- w158
              "RV Max Pressure" <- w157
              "RV RMS Pressure" <- w156
            }
            frame "Pitot (Pitot)" {
            }
            frame "Gen (Current)" {
              n63 = Multiply(x=w163, y=w164) -> (x*y=w162:dbl[])
              "Power" <- w162
              n64 = call-poly <vilib>:"RMS.vi"("X"=w162) -> ("rms value"=→"RMS Power":dbl)  [unwired: 1 out]
              "Current" <- w163
              "RMS Current" <- w160
              "Max Current" <- w159
            }
            frame "No Match", Default {
              n65 = One Button Dialog(message="Error in Signal Analysis", button name ("OK")="STOP") -> (true=w166:bool)
              n66 = Stop(stop? (T)=w166) -> ()
            }
          }
        }
      }
      frame "Build Results String" {
        n67 = local read "Results Files"() -> (w171:path[])
        n68 = for {
          N -> [w186]
          tunnel: w171 -> [w184] mode=indexing
          tunnel: w170 -> [w181]
          tunnel: w175 -> [w179]
          tunnel: w174 -> [w182]
          tunnel: w168 -> [w176]
          i -> [w178]
          n69 = Increment(x=w178) -> (x+1=w183:i32)
          n70 = Index Array(array=w181, index (row)=w178) -> (element=w180:dbl[])  [unwired: 1 in]
          n71 = Index Array(array=w179, index=w178) -> (element=w177:T5)
          n72 = Equal?(x=w186, y=w183) -> (x = y?=w185:bool)
          n73 = case shown="True" w185 {
            tunnel: w180 -> [w195 _]
            tunnel: w184 -> [w187 w213]
            tunnel: w177 -> [w194 _]
            tunnel: w182 -> [_ w211]
            tunnel: w176 -> [_ w207]
            frame False {
              n74 = Unbundle By Name(w194) -> ("Y"=w197:dbl)
              n75 = Number To Fractional String(number=w195, precision (6)=i16 7) -> (F-format string=w201:string[])  [unwired: 2 in]
              n76 = Number To Fractional String(number=w197, precision (6)=i16 7) -> (F-format string=w199:string)  [unwired: 2 in]
              n77 = Build Array (concatenate)(w199, w201, "") -> (w188:string[])
              n78 = for {
                shift-right: [w204] -> w192
                shift-left: "" -> [w205]
                tunnel: w188 -> [w203] mode=indexing
                n79 = Concatenate Strings(w205, w203, "\t") -> (w204:string)
              }
              n80 = Concatenate Strings(w192, "\r\n") -> (w193:string)
              n81 = call "Write_File_Simple.vi"("append to file? (new file:F)"=TRUE, "character string"=w193, "file path"=w187) -> ()  [unwired: 2 out]
            }
            frame True {
              w208 = ""
              n82 = local read "Zeros"() -> (w209:dbl[])
              n83 = local read "AS Freq"() -> (w210:dbl)
              n84 = Path To String(path=w211) -> (string=w206:string)
              n85 = Build Array (concatenate)(w210, w209) -> (w221:dbl[])
              n86 = for {
                tunnel: w221 -> [w230] mode=indexing
                shift-right: [w227] -> w220
                shift-left: string[] [] -> [w228]
                n87 = Number To Fractional String(number=w230, precision (6)=i16 7) -> (F-format string=w229:string)  [unwired: 2 in]
                n88 = Build Array (concatenate)(w228, w229, "") -> (w227:string[])
              }
              n89 = Build Array (concatenate)(w207, w208, w206, w208, w220) -> (w212:string[])
              n90 = for {
                shift-right: [w224] -> w215
                shift-left: "" -> [w225]
                tunnel: w212 -> [w223] mode=indexing
                n91 = Concatenate Strings(w225, w223, "\t") -> (w224:string)
              }
              n92 = Concatenate Strings(w215, "\r\n") -> (w214:string)
              n93 = call "Write_File_Simple.vi"("append to file? (new file:F)"=TRUE, "character string"=w214, "file path"=w213) -> ()  [unwired: 2 out]
            }
          }
        }
      }
      frame "Plot Data" {
        n94 = local read "AS Freq"() -> (w275:dbl)
        n95 = case shown="0, Default" w240 {
          tunnel: [w281 w283] -> w251
          tunnel: ["Velocity (m/s)" ("Plot.Plot Name") "Pressure (Pa)" ("Plot.Plot Name")] -> w239
          frame 1 {
            n96 = local read "Max Hot Wire"() -> (w281:dbl)
          }
          frame 0, Default {
            n97 = local read "RMS Pressure"() -> (w283:dbl)
          }
        }
        n98 = Reciprocal(x=w275) -> (1/x=w274:dbl)
        n99 = local read "Freq"() -> (w250:dbl)
        n100 = local read "Amp"() -> (w252:dbl)
        n101 = call-poly <vilib>:"Ramp Pattern.vi"("start"=0.0, "end"=w274, "samples"=w277) -> ("Ramp Pattern"=w266:dbl[])  [unwired: 7 in, 1 out]
        n102 = local read "Hotwire Velocity"() -> (w255:dbl[])
        n103 = Build Array(w250, w251, w252) -> (w249:dbl[])
        n104 = local read "Input Voltage"() -> (w257:dbl[])
        n105 = local read "Displacement"() -> (w256:dbl[])
        n106 = local read "Pressure"() -> (w254:dbl[])
        n107 = local read "Power"() -> (w237:dbl[])
        n108 = Build Array (concatenate)(w248, w249) -> (w247:dbl[][])
        n109 = Array Max & Min(array=w254) -> (max value=w259:dbl)  [unwired: 3 out]
        n110 = Array Max & Min(array=w266) -> (max value=w267:dbl)  [unwired: 3 out]
        n111 = Array Max & Min(array=w257) -> (max value=w265:dbl)  [unwired: 3 out]
        n112 = Array Max & Min(array=w256) -> (max value=w261:dbl)  [unwired: 3 out]
        n113 = Array Max & Min(array=w255) -> (max value=w263:dbl)  [unwired: 3 out]
        n114 = Array Max & Min(array=w237) -> (max value=w238:dbl)  [unwired: 3 out]
        n115 = Index Array(array=w247, index (col) #1=0 ("disabled index (col)"), index (col) #2=1 ("index (col)"), index (col) #3=2 ("index (col)")) -> (element #1=w243:dbl[], element #2=w242:dbl[])  [unwired: 3 in, 1 out]
        n116 = Divide(x=w254, y=w259) -> (x/y=w258:dbl[])
        n117 = Divide(x=w266, y=w267) -> (x/y=w236:dbl[])
        n118 = Divide(x=w257, y=w265) -> (x/y=w264:dbl[])
        n119 = Divide(x=w256, y=w261) -> (x/y=w260:dbl[])
        n120 = Divide(x=w255, y=w263) -> (x/y=w262:dbl[])
        n121 = Divide(x=w237, y=w238) -> (x/y=w235:dbl[])
        n122 = Bundle(w236, w258) -> (w271:cluster{dbl[], dbl[]})  [unwired: 1 in]
        n123 = Bundle(w236, w264) -> (w234:cluster{dbl[], dbl[]})  [unwired: 1 in]
        n124 = Bundle(w236, w260) -> (w272:cluster{dbl[], dbl[]})  [unwired: 1 in]
        n125 = Bundle(w236, w262) -> (w273:cluster{dbl[], dbl[]})  [unwired: 1 in]
        n126 = Bundle(w236, w235) -> (w233:cluster{dbl[], dbl[]})  [unwired: 1 in]
        n127 = Build Array(w234, w271) -> (→"Pressure":cluster{dbl[], dbl[]}[])
        n128 = Build Array(w234, w272) -> (→"Displacement":cluster{dbl[], dbl[]}[])
        n129 = Build Array(w234, w273) -> (→"Hot Wire":cluster{dbl[], dbl[]}[])
        n130 = Build Array(w234, w233) -> (→"Current Plot":cluster{dbl[], dbl[]}[])
        n131 = property on="Pressure v Frequency" class="XYGraph (strict)"("YScale.NameLbl.Text"=w239) -> ()  [unwired: 2 in, 2 out]
        n132 = Bundle(w243, w242) -> (→"Pressure v Frequency":cluster{dbl[], dbl[]})  [unwired: 1 in]
      }
      frame "End" {
        n133 = Strip Path(path=w299) -> (stripped path=w304:path)  [unwired: 1 out]
        n134 = Strip Path(path=w304) -> (stripped path=w302:path, name=w298:string)
        n135 = Strip Path(path=w302) -> (stripped path=w303:path)  [unwired: 1 out]
        n136 = Strip Path(path=w303) -> (stripped path=w301:path)  [unwired: 1 out]
        n137 = Concatenate Strings(w298, ".xls" ("string")) -> (w296:string)
        n138 = Build Path(base path=w301, name or relative path="Results_Post_Processed") -> (appended path=w295:path)
        n139 = Build Path(base path=w295, name or relative path=w296) -> (appended path=w294:path)
        n140 = Index Array(array=w290, index (col) #1=0 ("disabled index (col)"), index (col) #2=1 ("index (col)"), index (col) #3=2 ("index (col)")) -> (element #1=w286:dbl[], element #2=w288:dbl[], element #3=w285:dbl[])  [unwired: 3 in]
        n141 = call <vilib>:"Check if File or Folder Exists.vi"("path"=w294) -> ("file or folder exists?"=w289:bool, "dup path"=w287:path)  [unwired: 8 in, 1 out]
        n142 = case shown="True" w289 {
          tunnel: w288 -> [w310 w349]
          tunnel: w284 -> [w308 w347]
          tunnel: w287 -> [w319 w340]
          tunnel: w286 -> [w331 _]
          tunnel: w285 -> [w330 _]
          frame False {
            w328 = i16 7 ("precision (6)")
            n143 = Index Array(array=w330) -> (element=w329:dbl)  [unwired: 1 in]
            n144 = Number To Fractional String(number=w331, precision (6)=w328) -> (F-format string=w326:string[])  [unwired: 2 in]
            n145 = Number To Fractional String(number=w329, precision (6)=w328) -> (F-format string=w327:string)  [unwired: 2 in]
            n146 = Number To Fractional String(number=w310, precision (6)=i16 7) -> (F-format string=w317:string[])  [unwired: 2 in]
            n147 = Build Array (concatenate)(w327, w326) -> (w320:string[])
            n148 = Build Array (concatenate)(w308, w317) -> (w311:string[])
            n149 = for {
              shift-right: [w338] -> w324
              shift-left: "" -> [w339]
              tunnel: w320 -> [w337] mode=indexing
              n150 = Concatenate Strings(w339, w337, "\t") -> (w338:string)
            }
            n151 = for {
              shift-right: [w334] -> w315
              shift-left: "" -> [w335]
              tunnel: w311 -> [w333] mode=indexing
              n152 = Concatenate Strings(w335, w333, "\t") -> (w334:string)
            }
            n153 = Concatenate Strings(w324, "\r\n") -> (w325:string)
            n154 = Concatenate Strings(w315, "\r\n") -> (w316:string)
            n155 = call "Write_File_Simple.vi"("append to file? (new file:F)"=FALSE, "character string"=w325, "file path"=w319) -> ("file path Out"=w309:path)  [unwired: 1 out]
            n156 = call "Write_File_Simple.vi"("append to file? (new file:F)"=TRUE, "character string"=w316, "file path"=w309) -> ()  [unwired: 2 out]
          }
          frame True {
            n157 = Number To Fractional String(number=w349, precision (6)=i16 7) -> (F-format string=w348:string[])  [unwired: 2 in]
            n158 = Build Array (concatenate)(w347, w348) -> (w341:string[])
            n159 = for {
              shift-right: [w353] -> w345
              shift-left: "" -> [w354]
              tunnel: w341 -> [w352] mode=indexing
              n160 = Concatenate Strings(w354, w352, "\t") -> (w353:string)
            }
            n161 = Concatenate Strings(w345, "\r\n") -> (w346:string)
            n162 = call "Write_File_Simple.vi"("append to file? (new file:F)"=TRUE, "character string"=w346, "file path"=w340) -> ()  [unwired: 2 out]
          }
        }
      }
    }
  }
